vi "StatisticsOnFITSstacks.vi"() -> ()   [LabVIEW 2011]
panel:
  in  "file (use dialog)":path=path "C:/Users/christian/Desktop/tango-signaleSIM.txt"
  out "concatenated string":string="E:\\Auswertung_ISS\\data\\002_2018-06-21_16-44-14\\raw_I000_X0_C0.fits.SIM.fits, 1.293519E+0, 2.813395E+0, 3.203675E-2, 0.000000E+0, 5.713888E+2\r\nE:\\Auswertung_ISS\\data\\002_2018-06-21_16-44-14\\raw_I000_X0_C1.fits.SIM.fits, 5.156106E+0, 1.029898E+1, 3.548476E-1, 0.000000E+0, 1.040870E+3\r\nE:\\Auswertung_ISS\\data\\002_2018-06-21_16-44-14\\raw_I000_X0_C3.fits.SIM.fits, 4.121879E+0, 7.055258E+0, 2.127021E-1, 0.000000E+0, 5.426572E+2\r\nE:\\Auswertung_ISS\\data\\002_2018-06-21_16-44-14\\raw_I000_X1_C0.fits.SIM.fits, 1.210145E+0, 2.047290E+0, -9.516930E-3, 0.000000E+0, 2.892630E+2\r\nE:\\Auswertung_ISS\\data\\002_2018-06-21_16-44-14\\raw_I000_X1_C3.fits.SIM.fits, 1.346602E+0, 2.369957E+0, -2.971059E-2, 0.000000E+0, 2.189330E+2\r\nE:\\Auswertung_ISS\\data\\003_2018-07-03_15-08-29\\raw_I000_X0_C0.fits.SIM.fits, 1.338123E+0, 2.747078E+0, -2.947819E-2, 0.000000E+0, 9.794098E+2\r\nE:\\Auswertung_ISS\\data\\003_2018-07-03_15-08-29\\raw_I000_X0_C1.fits.SIM.fits, 3.859661E+0, 8.027792E+0, -2.797096E-1, 0.000000E+0, 7.325175E+2\r\nE:\\Auswertung_ISS\\data\\003_2018-07-03_15-08-29\\raw_I000_X0_C3.fits.SIM.fits, 2.238438E+0, 3.776091E+0, -1.215679E-1, 0.000000E+0, 6.079381E+2\r\nE:\\Auswertung_ISS\\data\\003_2018-07-03_15-08-29\\raw_I000_X1_C0.fits.SIM.fits, 1.522831E+0, 2.640957E+0, -6.579430E-3, 0.000000E+0, 7.584379E+2\r\nE:\\Auswertung_ISS\\data\\003_2018-07-03_15-08-29\\raw_I000_X1_C3.fits.SIM.fits, 1.066429E+0, 2.187258E+0, 8.379865E-3, 0.000000E+0, 5.129649E+2\r\nE:\\Auswertung_ISS\\data\\003_2018-07-03_15-08-29\\raw_I001_X1_C0.fits.SIM.fits, 1.376409E+0, 2.223739E+0, -6.037710E-3, 0.000000E+0, 5.685716E+2\r\nE:\\Auswertung_ISS\\data\\003_2018-07-03_15-08-29\\raw_I001_X1_C3.fits.SIM.fits, 9.524613E-1, 1.817422E+0, 4.163195E-3, 0.000000E+0, 6.636672E+2\r\nE:\\Auswertung_ISS\\data\\003_2018-07-03_15-08-29\\raw_I002_X1_C0.fits.SIM.fits, 1.321902E+0, 2.089704E+0, -8.378804E-3, 0.000000E+0, 7.800291E+2\r\nE:\\Auswertung_ISS\\data\\003_2018-07-03_15-08-29\\raw_I002_X1_C3.fits.SIM.fits, 9.022409E-1, 1.645853E+0, -5.385981E-3, 0.000000E+0, 8.949173E+2\r\nE:\\Auswertung_ISS\\data\\003_2018-07-03_15-08-29\\raw_I003_X1_C0.fits.SIM.fits, 1.288627E+0, 1.993243E+0, -1.267377E-2, 0.000000E+0, 5.885883E+2\r\nE:\\Auswertung_ISS\\data\\003_2018-07-03_15-08-29\\raw_I003_X1_C3.fits.SIM.fits, 8.580835E-1, 1.470445E+0, -1.397096E-2, 0.000000E+0, 1.369498E+3\r\nE:\\Auswertung_ISS\\data\\003_2018-07-03_15-08-29\\raw_I004_X1_C0.fits.SIM.fits, 1.244456E+0, 1.891138E+0, -1.474137E-2, 0.000000E+0, 8.155282E+2\r\nE:\\Auswertung_ISS\\data\\003_2018-07-03_15-08-29\\raw_I004_X1_C3.fits.SIM.fits, 7.920791E-1, 1.279965E+0, -1.287860E-2, 0.000000E+0, 9.381859E+2\r\nE:\\Auswertung_ISS\\data\\003_2018-07-03_15-08-29\\raw_I005_X1_C0.fits.SIM.fits, 1.217874E+0, 1.802349E+0, -1.420018E-2, 0.000000E+0, 7.741145E+2\r\nE:\\Auswertung_ISS\\data\\003_2018-07-03_15-08-29\\raw_I005_X1_C3.fits.SIM.fits, 7.460330E-1, 1.147673E+0, -9.173622E-3, 0.000000E+0, 6.827392E+2\r\nE:\\Auswertung_ISS\\data\\003_2018-07-03_15-08-29\\raw_I006_X1_C0.fits.SIM.fits, 1.196925E+0, 1.725176E+0, -1.303407E-2, 0.000000E+0, 3.640719E+2\r\nE:\\Auswertung_ISS\\data\\003_2018-07-03_15-08-29\\raw_I006_X1_C3.fits.SIM.fits, 7.214212E-1, 1.099456E+0, -7.464411E-3, 0.000000E+0, 2.052355E+3\r\nE:\\Auswertung_ISS\\data\\003_2018-07-03_15-08-29\\raw_I007_X1_C0.fits.SIM.fits, 1.184295E+0, 1.684428E+0, -1.213101E-2, 0.000000E+0, 3.740072E+2\r\nE:\\Auswertung_ISS\\data\\003_2018-07-03_15-08-29\\raw_I007_X1_C3.fits.SIM.fits, 7.082895E-1, 1.060245E+0, -6.374558E-3, 0.000000E+0, 1.029119E+3\r\nE:\\Auswertung_ISS\\data\\003_2018-07-03_15-08-29\\raw_I008_X1_C0.fits.SIM.fits, 1.178256E+0, 1.672969E+0, -1.182940E-2, 0.000000E+0, 7.563615E+2\r\nE:\\Auswertung_ISS\\data\\003_2018-07-03_15-08-29\\raw_I008_X1_C3.fits.SIM.fits, 7.006131E-1, 1.045075E+0, -5.954691E-3, 0.000000E+0, 1.337770E+3\r\nE:\\Auswertung_ISS\\data\\003_2018-07-03_15-08-29\\raw_I009_X0_C0.fits.SIM.fits, 1.216490E+0, 2.542340E+0, -2.450155E-2, 0.000000E+0, 7.565395E+2\r\nE:\\Auswertung_ISS\\data\\003_2018-07-03_15-08-29\\raw_I009_X0_C1.fits.SIM.fits, 3.969645E+0, 8.299880E+0, -3.314994E-1, 0.000000E+0, 9.914262E+2\r\nE:\\Auswertung_ISS\\data\\003_2018-07-03_15-08-29\\raw_I009_X0_C3.fits.SIM.fits, 1.936800E+0, 3.176954E+0, -1.136370E-1, 0.000000E+0, 6.554843E+2\r\nE:\\Auswertung_ISS\\data\\003_2018-07-03_15-08-29\\raw_I009_X1_C0.fits.SIM.fits, 1.151698E+2, 2.053238E+3, 6.473798E+1, 0.000000E+0, 4.964122E+6\r\nE:\\Auswertung_ISS\\data\\003_2018-07-03_15-08-29\\raw_I009_X1_C3.fits.SIM.fits, 1.220527E+3, 1.606567E+4, 6.178774E+2, 0.000000E+0, 2.381387E+7\r\nE:\\Auswertung_ISS\\data\\004_2018-07-03_17-33-15\\raw_I000_X0_C0.fits.SIM.fits, 1.178057E+0, 2.387788E+0, -2.293336E-2, 0.000000E+0, 3.530892E+2\r\nE:\\Auswertung_ISS\\data\\004_2018-07-03_17-33-15\\raw_I000_X0_C1.fits.SIM.fits, 3.207769E+0, 6.773418E+0, -1.955297E-1, 0.000000E+0, 1.686196E+3\r\nE:\\Auswertung_ISS\\data\\004_2018-07-03_17-33-15\\raw_I000_X0_C3.fits.SIM.fits, 1.521199E+0, 2.480720E+0, -5.475838E-2, 0.000000E+0, 3.812462E+2\r\nE:\\Auswertung_ISS\\data\\004_2018-07-03_17-33-15\\raw_I000_X1_C0.fits.SIM.fits, 1.207292E+0, 1.949696E+0, -5.863263E-3, 0.000000E+0, 8.527518E+2\r\nE:\\Auswertung_ISS\\data\\004_2018-07-03_17-33-15\\raw_I000_X1_C3.fits.SIM.fits, 7.241709E-1, 1.295861E+0, 8.837919E-4, 0.000000E+0, 1.748222E+3\r\nE:\\Auswertung_ISS\\data\\004_2018-07-03_17-33-15\\raw_I001_X1_C0.fits.SIM.fits, 1.169572E+0, 1.829014E+0, -5.958593E-3, 0.000000E+0, 5.068069E+2\r\nE:\\Auswertung_ISS\\data\\004_2018-07-03_17-33-15\\raw_I001_X1_C3.fits.SIM.fits, 7.097706E-1, 1.163805E+0, -2.180760E-4, 0.000000E+0, 1.272369E+3\r\nE:\\Auswertung_ISS\\data\\004_2018-07-03_17-33-15\\raw_I002_X1_C0.fits.SIM.fits, 1.153690E+0, 1.775655E+0, -6.165336E-3, 0.000000E+0, 8.572842E+2\r\nE:\\Auswertung_ISS\\data\\004_2018-07-03_17-33-15\\raw_I002_X1_C3.fits.SIM.fits, 6.968903E-1, 1.093959E+0, -9.725231E-4, 0.000000E+0, 5.995302E+2\r\nE:\\Auswertung_ISS\\data\\004_2018-07-03_17-33-15\\raw_I003_X1_C0.fits.SIM.fits, 1.143082E+0, 1.745283E+0, -6.109823E-3, 0.000000E+0, 8.502672E+2\r\nE:\\Auswertung_ISS\\data\\004_2018-07-03_17-33-15\\raw_I003_X1_C3.fits.SIM.fits, 6.854192E-1, 1.067064E+0, -1.198857E-3, 0.000000E+0, 6.685107E+2\r\nE:\\Auswertung_ISS\\data\\004_2018-07-03_17-33-15\\raw_I004_X1_C0.fits.SIM.fits, 1.133617E+0, 1.709983E+0, -6.070233E-3, 0.000000E+0, 5.567000E+2\r\nE:\\Auswertung_ISS\\data\\004_2018-07-03_17-33-15\\raw_I004_X1_C3.fits.SIM.fits, 6.757222E-1, 1.036550E+0, -1.148639E-3, 0.000000E+0, 8.245127E+2\r\nE:\\Auswertung_ISS\\data\\004_2018-07-03_17-33-15\\raw_I005_X1_C0.fits.SIM.fits, 1.124385E+0, 1.650913E+0, -6.445620E-3, 0.000000E+0, 1.047790E+3\r\nE:\\Auswertung_ISS\\data\\004_2018-07-03_17-33-15\\raw_I005_X1_C3.fits.SIM.fits, 6.672083E-1, 1.008144E+0, -1.706395E-3, 0.000000E+0, 1.310684E+3\r\nE:\\Auswertung_ISS\\data\\004_2018-07-03_17-33-15\\raw_I006_X1_C0.fits.SIM.fits, 1.118813E+0, 1.641358E+0, -6.489867E-3, 0.000000E+0, 5.621022E+2\r\nE:\\Auswertung_ISS\\data\\004_2018-07-03_17-33-15\\raw_I006_X1_C3.fits.SIM.fits, 6.614291E-1, 9.921280E-1, -1.909784E-3, 0.000000E+0, 1.047368E+3\r\nE:\\Auswertung_ISS\\data\\004_2018-07-03_17-33-15\\raw_I007_X1_C0.fits.SIM.fits, 1.113078E+0, 1.626524E+0, -6.676457E-3, 0.000000E+0, 6.429068E+2\r\nE:\\Auswertung_ISS\\data\\004_2018-07-03_17-33-15\\raw_I007_X1_C3.fits.SIM.fits, 6.557754E-1, 9.745117E-1, -2.120740E-3, 0.000000E+0, 7.079556E+2\r\nE:\\Auswertung_ISS\\data\\004_2018-07-03_17-33-15\\raw_I008_X1_C0.fits.SIM.fits, 1.106670E+0, 1.609972E+0, -6.478068E-3, 0.000000E+0, 5.270333E+2\r\nE:\\Auswertung_ISS\\data\\004_2018-07-03_17-33-15\\raw_I008_X1_C3.fits.SIM.fits, 6.534819E-1, 9.693815E-1, -1.453581E-3, 0.000000E+0, 6.050910E+2\r\nE:\\Auswertung_ISS\\data\\004_2018-07-03_17-33-15\\raw_I009_X1_C0.fits.SIM.fits, 1.103888E+0, 1.608102E+0, -6.673347E-3, 0.000000E+0, 7.272290E+2\r\nE:\\Auswertung_ISS\\data\\004_2018-07-03_17-33-15\\raw_I009_X1_C3.fits.SIM.fits, 6.520411E-1, 9.801836E-1, -1.973502E-3, 0.000000E+0, 7.507390E+2\r\nE:\\Auswertung_ISS\\data\\004_2018-07-03_17-33-15\\raw_I010_X1_C0.fits.SIM.fits, 1.099766E+0, 1.593314E+0, -6.739226E-3, 0.000000E+0, 6.720167E+2\r\nE:\\Auswertung_ISS\\data\\004_2018-07-03_17-33-15\\raw_I010_X1_C3.fits.SIM.fits, 6.444918E-1, 9.767788E-1, -1.939564E-3, 0.000000E+0, 6.929294E+2\r\nE:\\Auswertung_ISS\\data\\004_2018-07-03_17-33-15\\raw_I011_X1_C0.fits.SIM.fits, 1.098232E+0, 1.590663E+0, -6.803889E-3, 0.000000E+0, 6.297327E+2\r\nE:\\Auswertung_ISS\\data\\004_2018-07-03_17-33-15\\raw_I011_X1_C3.fits.SIM.fits, 6.416938E-1, 9.659073E-1, -2.201290E-3, 0.000000E+0, 1.132601E+3\r\nE:\\Auswertung_ISS\\data\\004_2018-07-03_17-33-15\\raw_I012_X1_C0.fits.SIM.fits, 1.094868E+0, 1.581222E+0, -6.771624E-3, 0.000000E+0, 6.924265E+2\r\nE:\\Auswertung_ISS\\data\\004_2018-07-03_17-33-15\\raw_I012_X1_C3.fits.SIM.fits, 6.348257E-1, 9.330733E-1, -2.023490E-3, 0.000000E+0, 1.007330E+3\r\nE:\\Auswertung_ISS\\data\\004_2018-07-03_17-33-15\\raw_I013_X1_C0.fits.SIM.fits, 1.091418E+0, 1.572815E+0, -6.660544E-3, 0.000000E+0, 8.789351E+2\r\nE:\\Auswertung_ISS\\data\\004_2018-07-03_17-33-15\\raw_I013_X1_C3.fits.SIM.fits, 6.288961E-1, 9.195451E-1, -1.885985E-3, 0.000000E+0, 1.165087E+3\r\nE:\\Auswertung_ISS\\data\\004_2018-07-03_17-33-15\\raw_I014_X1_C0.fits.SIM.fits, 1.088608E+0, 1.572637E+0, -6.572176E-3, 0.000000E+0, 7.930138E+2\r\nE:\\Auswertung_ISS\\data\\004_2018-07-03_17-33-15\\raw_I014_X1_C3.fits.SIM.fits, 6.240145E-1, 9.116531E-1, -1.725730E-3, 0.000000E+0, 9.153251E+2\r\nE:\\Auswertung_ISS\\data\\004_2018-07-03_17-33-15\\raw_I015_X1_C0.fits.SIM.fits, 1.084505E+0, 1.558305E+0, -6.505683E-3, 0.000000E+0, 4.014997E+2\r\nE:\\Auswertung_ISS\\data\\004_2018-07-03_17-33-15\\raw_I015_X1_C3.fits.SIM.fits, 6.178792E-1, 9.008335E-1, -1.617021E-3, 0.000000E+0, 1.074420E+3\r\nE:\\Auswertung_ISS\\data\\004_2018-07-03_17-33-15\\raw_I016_X1_C0.fits.SIM.fits, 1.083422E+0, 1.556624E+0, -6.624974E-3, 0.000000E+0, 3.853266E+2\r\nE:\\Auswertung_ISS\\data\\004_2018-07-03_17-33-15\\raw_I016_X1_C3.fits.SIM.fits, 6.142787E-1, 9.021998E-1, -1.622850E-3, 0.000000E+0, 8.832935E+2\r\nE:\\Auswertung_ISS\\data\\004_2018-07-03_17-33-15\\raw_I017_X1_C0.fits.SIM.fits, 1.241818E+0, 1.898849E+0, -1.011896E-2, 0.000000E+0, 6.071580E+2\r\nE:\\Auswertung_ISS\\data\\004_2018-07-03_17-33-15\\raw_I017_X1_C3.fits.SIM.fits, 6.135428E-1, 9.080176E-1, -2.219069E-3, 0.000000E+0, 1.471575E+3\r\nE:\\Auswertung_ISS\\data\\005_2018-07-04_08-02-54\\raw_I000_X0_C0.fits.SIM.fits, 1.168267E+0, 2.392403E+0, -2.321325E-2, 0.000000E+0, 5.743918E+2\r\nE:\\Auswertung_ISS\\data\\005_2018-07-04_08-02-54\\raw_I000_X0_C1.fits.SIM.fits, 3.042382E+0, 6.318101E+0, -1.780247E-1, 0.000000E+0, 1.179049E+3\r\nE:\\Auswertung_ISS\\data\\005_2018-07-04_08-02-54\\raw_I000_X0_C3.fits.SIM.fits, 1.098923E+0, 1.709743E+0, -2.960586E-2, 0.000000E+0, 3.829828E+2\r\nE:\\Auswertung_ISS\\data\\005_2018-07-04_08-02-54\\raw_I000_X1_C0.fits.SIM.fits, 1.228053E+0, 1.853084E+0, -9.042175E-3, 0.000000E+0, 4.665842E+2\r\nE:\\Auswertung_ISS\\data\\005_2018-07-04_08-02-54\\raw_I000_X1_C3.fits.SIM.fits, 5.740621E-1, 8.157131E-1, -1.532513E-3, 0.000000E+0, 9.479493E+2\r\nE:\\Auswertung_ISS\\data\\005_2018-07-04_08-02-54\\raw_I001_X1_C0.fits.SIM.fits, 1.166965E+0, 1.716451E+0, -7.717278E-3, 0.000000E+0, 1.209727E+3\r\nE:\\Auswertung_ISS\\data\\005_2018-07-04_08-02-54\\raw_I001_X1_C3.fits.SIM.fits, 5.649782E-1, 8.012455E-1, -1.272490E-3, 0.000000E+0, 1.392420E+3\r\nE:\\Auswertung_ISS\\data\\005_2018-07-04_08-02-54\\raw_I002_X1_C0.fits.SIM.fits, 1.147424E+0, 1.703185E+0, -7.049788E-3, 0.000000E+0, 4.221453E+2\r\nE:\\Auswertung_ISS\\data\\005_2018-07-04_08-02-54\\raw_I002_X1_C3.fits.SIM.fits, 5.609546E-1, 7.931188E-1, -1.130987E-3, 0.000000E+0, 9.405351E+2\r\nE:\\Auswertung_ISS\\data\\005_2018-07-04_08-02-54\\raw_I003_X1_C0.fits.SIM.fits, 1.126167E+0, 1.636829E+0, -7.009850E-3, 0.000000E+0, 7.209102E+2\r\nE:\\Auswertung_ISS\\data\\005_2018-07-04_08-02-54\\raw_I003_X1_C3.fits.SIM.fits, 5.537584E-1, 7.808799E-1, -7.431867E-4, 0.000000E+0, 1.088224E+3\r\nE:\\Auswertung_ISS\\data\\005_2018-07-04_08-02-54\\raw_I004_X1_C0.fits.SIM.fits, 1.113321E+0, 1.610422E+0, -6.982198E-3, 0.000000E+0, 3.967598E+2\r\nE:\\Auswertung_ISS\\data\\005_2018-07-04_08-02-54\\raw_I004_X1_C3.fits.SIM.fits, 5.514046E-1, 7.721213E-1, -7.544226E-4, 0.000000E+0, 8.216857E+2\r\nE:\\Auswertung_ISS\\data\\005_2018-07-04_08-02-54\\raw_I005_X1_C0.fits.SIM.fits, 1.103067E+0, 1.593565E+0, -6.857917E-3, 0.000000E+0, 4.775246E+2\r\nE:\\Auswertung_ISS\\data\\005_2018-07-04_08-02-54\\raw_I005_X1_C3.fits.SIM.fits, 5.486360E-1, 7.665561E-1, -6.179845E-4, 0.000000E+0, 5.884370E+2\r\nE:\\Auswertung_ISS\\data\\005_2018-07-04_08-02-54\\raw_I006_X1_C0.fits.SIM.fits, 1.093904E+0, 1.570558E+0, -6.920714E-3, 0.000000E+0, 6.544910E+2\r\nE:\\Auswertung_ISS\\data\\005_2018-07-04_08-02-54\\raw_I006_X1_C3.fits.SIM.fits, 5.464946E-1, 7.668871E-1, -6.099782E-4, 0.000000E+0, 1.330119E+3\r\nE:\\Auswertung_ISS\\data\\005_2018-07-04_08-02-54\\raw_I007_X1_C0.fits.SIM.fits, 1.087188E+0, 1.564195E+0, -6.751027E-3, 0.000000E+0, 5.254551E+2\r\nE:\\Auswertung_ISS\\data\\005_2018-07-04_08-02-54\\raw_I007_X1_C3.fits.SIM.fits, 5.451777E-1, 7.614440E-1, -5.663460E-4, 0.000000E+0, 9.518828E+2\r\nE:\\Auswertung_ISS\\data\\005_2018-07-04_08-02-54\\raw_I008_X1_C0.fits.SIM.fits, 1.079745E+0, 1.542835E+0, -6.759820E-3, 0.000000E+0, 4.754071E+2\r\nE:\\Auswertung_ISS\\data\\005_2018-07-04_08-02-54\\raw_I008_X1_C3.fits.SIM.fits, 5.436806E-1, 7.669905E-1, -6.040051E-4, 0.000000E+0, 1.077933E+3\r\nE:\\Auswertung_ISS\\data\\005_2018-07-04_08-02-54\\raw_I009_X1_C0.fits.SIM.fits, 1.075054E+0, 1.537219E+0, -6.715304E-3, 0.000000E+0, 1.070141E+3\r\nE:\\Auswertung_ISS\\data\\005_2018-07-04_08-02-54\\raw_I009_X1_C3.fits.SIM.fits, 5.419445E-1, 7.547276E-1, -6.042233E-4, 0.000000E+0, 1.172648E+3\r\nE:\\Auswertung_ISS\\data\\005_2018-07-04_08-02-54\\raw_I010_X1_C0.fits.SIM.fits, 1.071120E+0, 1.528894E+0, -6.637398E-3, 0.000000E+0, 6.953884E+2\r\nE:\\Auswertung_ISS\\data\\005_2018-07-04_08-02-54\\raw_I010_X1_C3.fits.SIM.fits, 5.398463E-1, 7.559122E-1, -5.406494E-4, 0.000000E+0, 1.200631E+3\r\nE:\\Auswertung_ISS\\data\\005_2018-07-04_08-02-54\\raw_I011_X1_C0.fits.SIM.fits, 1.066154E+0, 1.515149E+0, -6.609291E-3, 0.000000E+0, 4.025648E+2\r\nE:\\Auswertung_ISS\\data\\005_2018-07-04_08-02-54\\raw_I011_X1_C3.fits.SIM.fits, 5.381187E-1, 7.581280E-1, -4.396083E-4, 0.000000E+0, 1.214015E+3\r\nE:\\Auswertung_ISS\\data\\005_2018-07-04_08-02-54\\raw_I012_X1_C0.fits.SIM.fits, 1.062224E+0, 1.514587E+0, -6.448907E-3, 0.000000E+0, 6.856676E+2\r\nE:\\Auswertung_ISS\\data\\005_2018-07-04_08-02-54\\raw_I012_X1_C3.fits.SIM.fits, 5.366250E-1, 7.576223E-1, -3.866185E-4, 0.000000E+0, 1.015641E+3\r\nE:\\Auswertung_ISS\\data\\005_2018-07-04_08-02-54\\raw_I013_X1_C0.fits.SIM.fits, 1.057811E+0, 1.501086E+0, -6.549502E-3, 0.000000E+0, 8.431631E+2\r\nE:\\Auswertung_ISS\\data\\005_2018-07-04_08-02-54\\raw_I013_X1_C3.fits.SIM.fits, 5.350741E-1, 7.434772E-1, -3.976152E-4, 0.000000E+0, 1.028520E+3\r\nE:\\Auswertung_ISS\\data\\005_2018-07-04_08-02-54\\raw_I014_X1_C0.fits.SIM.fits, 1.055553E+0, 1.498822E+0, -6.397800E-3, 0.000000E+0, 5.896923E+2\r\nE:\\Auswertung_ISS\\data\\005_2018-07-04_08-02-54\\raw_I014_X1_C3.fits.SIM.fits, 5.333580E-1, 7.450038E-1, -3.825911E-4, 0.000000E+0, 9.034543E+2\r\nE:\\Auswertung_ISS\\data\\005_2018-07-04_08-02-54\\raw_I015_X1_C0.fits.SIM.fits, 1.051548E+0, 1.486582E+0, -6.435934E-3, 0.000000E+0, 2.464364E+2\r\nE:\\Auswertung_ISS\\data\\005_2018-07-04_08-02-54\\raw_I015_X1_C3.fits.SIM.fits, 5.313362E-1, 7.351835E-1, -3.081133E-4, 0.000000E+0, 8.765760E+2\r\nE:\\Auswertung_ISS\\data\\005_2018-07-04_08-02-54\\raw_I016_X1_C0.fits.SIM.fits, 1.047979E+0, 1.483462E+0, -6.301912E-3, 0.000000E+0, 4.212937E+2\r\nE:\\Auswertung_ISS\\data\\005_2018-07-04_08-02-54\\raw_I016_X1_C3.fits.SIM.fits, 5.303586E-1, 7.424460E-1, -3.963325E-4, 0.000000E+0, 1.428170E+3\r\nE:\\Auswertung_ISS\\data\\006_2018-07-04_15-43-18\\raw_I000_X0_C0.fits.SIM.fits, 1.173188E+0, 2.418540E+0, -2.354629E-2, 0.000000E+0, 4.402941E+2\r\nE:\\Auswertung_ISS\\data\\006_2018-07-04_15-43-18\\raw_I000_X0_C1.fits.SIM.fits, 2.924494E+0, 6.028345E+0, -1.636071E-1, 0.000000E+0, 9.315766E+2\r\nE:\\Auswertung_ISS\\data\\006_2018-07-04_15-43-18\\raw_I000_X0_C3.fits.SIM.fits, 9.369917E-1, 1.419599E+0, -1.991960E-2, 0.000000E+0, 6.888892E+2\r\nE:\\Auswertung_ISS\\data\\006_2018-07-04_15-43-18\\raw_I000_X1_C0.fits.SIM.fits, 1.167226E+0, 1.601891E+0, -1.181800E-2, 0.000000E+0, 5.933480E+2\r\nE:\\Auswertung_ISS\\data\\006_2018-07-04_15-43-18\\raw_I000_X1_C3.fits.SIM.fits, 5.161158E-1, 7.151016E-1, -4.825938E-4, 0.000000E+0, 1.697749E+3\r\nE:\\Auswertung_ISS\\data\\006_2018-07-04_15-43-18\\raw_I001_X1_C0.fits.SIM.fits, 1.116488E+0, 1.530844E+0, -9.946897E-3, 0.000000E+0, 6.367750E+2\r\nE:\\Auswertung_ISS\\data\\006_2018-07-04_15-43-18\\raw_I001_X1_C3.fits.SIM.fits, 5.154800E-1, 7.122431E-1, -6.673413E-4, 0.000000E+0, 1.607819E+3\r\nE:\\Auswertung_ISS\\data\\006_2018-07-04_15-43-18\\raw_I002_X1_C0.fits.SIM.fits, 1.098814E+0, 1.505064E+0, -9.540462E-3, 0.000000E+0, 2.874549E+2\r\nE:\\Auswertung_ISS\\data\\006_2018-07-04_15-43-18\\raw_I002_X1_C3.fits.SIM.fits, 5.132112E-1, 7.099640E-1, -5.868003E-4, 0.000000E+0, 1.146126E+3\r\nE:\\Auswertung_ISS\\data\\006_2018-07-04_15-43-18\\raw_I003_X1_C0.fits.SIM.fits, 1.087255E+0, 1.488291E+0, -9.129129E-3, 0.000000E+0, 3.591404E+2\r\nE:\\Auswertung_ISS\\data\\006_2018-07-04_15-43-18\\raw_I003_X1_C3.fits.SIM.fits, 5.118757E-1, 7.201306E-1, -5.091988E-4, 0.000000E+0, 1.603813E+3\r\nE:\\Auswertung_ISS\\data\\007_2018-07-04_16-44-22\\raw_I000_X0_C0.fits.SIM.fits, 1.153519E+0, 2.645130E+0, 2.393591E-2, 0.000000E+0, 3.971248E+2\r\nE:\\Auswertung_ISS\\data\\007_2018-07-04_16-44-22\\raw_I000_X0_C1.fits.SIM.fits, 3.857970E+0, 7.510054E+0, 6.305399E-2, 0.000000E+0, 9.667203E+2\r\nE:\\Auswertung_ISS\\data\\007_2018-07-04_16-44-22\\raw_I000_X0_C3.fits.SIM.fits, 1.023600E+0, 1.481754E+0, 4.806154E-3, 0.000000E+0, 2.218139E+2\r\nE:\\Auswertung_ISS\\data\\007_2018-07-04_16-44-22\\raw_I000_X1_C0.fits.SIM.fits, 1.196240E+0, 1.789233E+0, -7.721109E-3, 0.000000E+0, 2.244067E+2\r\nE:\\Auswertung_ISS\\data\\007_2018-07-04_16-44-22\\raw_I000_X1_C3.fits.SIM.fits, 5.829489E-1, 8.366924E-1, -8.507837E-4, 0.000000E+0, 9.379310E+2\r\nE:\\Auswertung_ISS\\data\\007_2018-07-04_16-44-22\\raw_I001_X1_C0.fits.SIM.fits, 1.138294E+0, 1.672213E+0, -6.483374E-3, 0.000000E+0, 5.219246E+2\r\nE:\\Auswertung_ISS\\data\\007_2018-07-04_16-44-22\\raw_I001_X1_C3.fits.SIM.fits, 5.742043E-1, 8.091986E-1, -7.224752E-4, 0.000000E+0, 6.994556E+2\r\nE:\\Auswertung_ISS\\data\\007_2018-07-04_16-44-22\\raw_I002_X1_C0.fits.SIM.fits, 1.117667E+0, 1.610874E+0, -5.967891E-3, 0.000000E+0, 6.300037E+2\r\nE:\\Auswertung_ISS\\data\\007_2018-07-04_16-44-22\\raw_I002_X1_C3.fits.SIM.fits, 5.677322E-1, 7.945078E-1, -4.561589E-4, 0.000000E+0, 6.261265E+2\r\nE:\\Auswertung_ISS\\data\\007_2018-07-04_16-44-22\\raw_I003_X1_C0.fits.SIM.fits, 1.104924E+0, 1.613847E+0, -5.905481E-3, 0.000000E+0, 6.381712E+2\r\nE:\\Auswertung_ISS\\data\\007_2018-07-04_16-44-22\\raw_I003_X1_C3.fits.SIM.fits, 5.665135E-1, 8.095917E-1, -4.370291E-4, 0.000000E+0, 9.460343E+2\r\nE:\\Auswertung_ISS\\data\\007_2018-07-04_16-44-22\\raw_I004_X1_C0.fits.SIM.fits, 1.094761E+0, 1.586387E+0, -5.725719E-3, 0.000000E+0, 4.823523E+2\r\nE:\\Auswertung_ISS\\data\\007_2018-07-04_16-44-22\\raw_I004_X1_C3.fits.SIM.fits, 5.646007E-1, 8.049347E-1, -3.713122E-4, 0.000000E+0, 9.834833E+2\r\nE:\\Auswertung_ISS\\data\\007_2018-07-04_16-44-22\\raw_I005_X1_C0.fits.SIM.fits, 1.086430E+0, 1.550623E+0, -5.757585E-3, 0.000000E+0, 7.921680E+2\r\nE:\\Auswertung_ISS\\data\\007_2018-07-04_16-44-22\\raw_I005_X1_C3.fits.SIM.fits, 5.622428E-1, 7.931760E-1, -1.688326E-4, 0.000000E+0, 1.029930E+3\r\nE:\\Auswertung_ISS\\data\\007_2018-07-04_16-44-22\\raw_I006_X1_C0.fits.SIM.fits, 1.080670E+0, 1.556944E+0, -5.527289E-3, 0.000000E+0, 4.178517E+2\r\nE:\\Auswertung_ISS\\data\\007_2018-07-04_16-44-22\\raw_I006_X1_C3.fits.SIM.fits, 5.617751E-1, 7.960590E-1, -7.710413E-5, 0.000000E+0, 9.626111E+2\r\nE:\\Auswertung_ISS\\data\\007_2018-07-04_16-44-22\\raw_I007_X1_C0.fits.SIM.fits, 1.073678E+0, 1.525147E+0, -5.556067E-3, 0.000000E+0, 5.914534E+2\r\nE:\\Auswertung_ISS\\data\\007_2018-07-04_16-44-22\\raw_I007_X1_C3.fits.SIM.fits, 5.592173E-1, 7.789348E-1, -4.470449E-6, 0.000000E+0, 5.747207E+2\r\nE:\\Auswertung_ISS\\data\\007_2018-07-04_16-44-22\\raw_I008_X1_C0.fits.SIM.fits, 1.070393E+0, 1.532612E+0, -5.517926E-3, 0.000000E+0, 6.460666E+2\r\nE:\\Auswertung_ISS\\data\\007_2018-07-04_16-44-22\\raw_I008_X1_C3.fits.SIM.fits, 5.584064E-1, 7.797402E-1, -1.403181E-5, 0.000000E+0, 4.066313E+2\r\nE:\\Auswertung_ISS\\data\\007_2018-07-04_16-44-22\\raw_I008_X1_C3.fits.simpleSIM.fits, 9.756062E-1, 5.934669E-1, -1.062698E-3, 3.518001E-2, 4.811809E+2\r\nE:\\Auswertung_ISS\\data\\007_2018-07-04_16-44-22\\raw_I009_X1_C0.fits.SIM.fits, 1.064844E+0, 1.507894E+0, -5.596534E-3, 0.000000E+0, 4.210096E+2\r\nE:\\Auswertung_ISS\\data\\007_2018-07-04_16-44-22\\raw_I009_X1_C3.fits.SIM.fits, 5.560395E-1, 7.785271E-1, -1.746596E-5, 0.000000E+0, 1.219767E+3\r\nE:\\Auswertung_ISS\\data\\007_2018-07-04_16-44-22\\raw_I010_X1_C0.fits.SIM.fits, 1.062220E+0, 1.504640E+0, -5.459205E-3, 0.000000E+0, 6.228591E+2\r\nE:\\Auswertung_ISS\\data\\007_2018-07-04_16-44-22\\raw_I010_X1_C3.fits.SIM.fits, 5.553953E-1, 7.835472E-1, 5.496466E-5, 0.000000E+0, 1.274058E+3\r\nE:\\Auswertung_ISS\\data\\007_2018-07-04_16-44-22\\raw_I011_X1_C0.fits.SIM.fits, 1.060179E+0, 1.500548E+0, -5.420390E-3, 0.000000E+0, 4.995820E+2\r\nE:\\Auswertung_ISS\\data\\007_2018-07-04_16-44-22\\raw_I011_X1_C3.fits.SIM.fits, 5.544396E-1, 7.838519E-1, 2.043480E-4, 0.000000E+0, 1.140602E+3\r\nE:\\Auswertung_ISS\\data\\007_2018-07-04_16-44-22\\raw_I012_X1_C0.fits.SIM.fits, 1.056946E+0, 1.491268E+0, -5.362876E-3, 0.000000E+0, 3.350965E+2\r\nE:\\Auswertung_ISS\\data\\007_2018-07-04_16-44-22\\raw_I012_X1_C3.fits.SIM.fits, 5.532384E-1, 7.741418E-1, 2.192681E-4, 0.000000E+0, 9.582665E+2\r\nE:\\Auswertung_ISS\\data\\007_2018-07-04_16-44-22\\raw_I013_X1_C0.fits.SIM.fits, 1.054764E+0, 1.495314E+0, -5.343243E-3, 0.000000E+0, 3.678161E+2\r\nE:\\Auswertung_ISS\\data\\007_2018-07-04_16-44-22\\raw_I013_X1_C3.fits.SIM.fits, 5.516079E-1, 7.765394E-1, 1.682077E-4, 0.000000E+0, 1.040956E+3\r\nE:\\Auswertung_ISS\\data\\007_2018-07-04_16-44-22\\raw_I014_X1_C0.fits.SIM.fits, 1.051305E+0, 1.483902E+0, -5.243355E-3, 0.000000E+0, 5.850872E+2\r\nE:\\Auswertung_ISS\\data\\007_2018-07-04_16-44-22\\raw_I014_X1_C3.fits.SIM.fits, 5.500311E-1, 7.715969E-1, 2.253367E-4, 0.000000E+0, 1.121011E+3\r\nE:\\Auswertung_ISS\\data\\007_2018-07-04_16-44-22\\raw_I015_X1_C0.fits.SIM.fits, 1.047873E+0, 1.477831E+0, -5.204884E-3, 0.000000E+0, 4.423718E+2\r\nE:\\Auswertung_ISS\\data\\007_2018-07-04_16-44-22\\raw_I015_X1_C3.fits.SIM.fits, 5.480902E-1, 7.653563E-1, 2.163062E-4, 0.000000E+0, 1.302920E+3\r\nE:\\Auswertung_ISS\\data\\007_2018-07-04_16-44-22\\raw_I016_X1_C0.fits.SIM.fits, 1.047071E+0, 1.487131E+0, -5.224378E-3, 0.000000E+0, 9.012682E+2\r\nE:\\Auswertung_ISS\\data\\007_2018-07-04_16-44-22\\raw_I016_X1_C3.fits.SIM.fits, 5.473597E-1, 7.600744E-1, 1.331081E-4, 0.000000E+0, 5.495349E+2\r\nE:\\Auswertung_ISS\\data\\007_2018-07-04_16-44-22\\raw_I017_X1_C0.fits.SIM.fits, 1.162750E+0, 1.656961E+0, -8.553688E-3, 0.000000E+0, 4.017816E+2\r\nE:\\Auswertung_ISS\\data\\007_2018-07-04_16-44-22\\raw_I017_X1_C3.fits.SIM.fits, 5.456086E-1, 7.595779E-1, -2.192173E-4, 0.000000E+0, 1.091998E+3\r\nE:\\Auswertung_ISS\\data\\008_2018-07-05_08-02-52\\raw_I000_X0_C0.fits.SIM.fits, 1.148379E+0, 2.222971E+0, -1.844273E-2, 0.000000E+0, 3.856597E+2\r\nE:\\Auswertung_ISS\\data\\008_2018-07-05_08-02-52\\raw_I000_X0_C1.fits.SIM.fits, 2.394992E+0, 4.660775E+0, -7.314335E-2, 0.000000E+0, 7.939623E+2\r\nE:\\Auswertung_ISS\\data\\008_2018-07-05_08-02-52\\raw_I000_X0_C3.fits.SIM.fits, 7.212795E-1, 1.039594E+0, -5.723648E-3, 0.000000E+0, 4.026962E+2\r\nE:\\Auswertung_ISS\\data\\008_2018-07-05_08-02-52\\raw_I000_X1_C0.fits.SIM.fits, 1.202009E+0, 1.771153E+0, -8.815809E-3, 0.000000E+0, 4.285009E+2\r\nE:\\Auswertung_ISS\\data\\008_2018-07-05_08-02-52\\raw_I000_X1_C3.fits.SIM.fits, 5.883181E-1, 8.647142E-1, -1.495725E-3, 0.000000E+0, 8.403303E+2\r\nE:\\Auswertung_ISS\\data\\008_2018-07-05_08-02-52\\raw_I001_X1_C0.fits.SIM.fits, 1.141505E+0, 1.658387E+0, -7.034378E-3, 0.000000E+0, 5.092637E+2\r\nE:\\Auswertung_ISS\\data\\008_2018-07-05_08-02-52\\raw_I001_X1_C3.fits.SIM.fits, 5.780757E-1, 8.329380E-1, -1.291502E-3, 0.000000E+0, 7.277889E+2\r\nE:\\Auswertung_ISS\\data\\008_2018-07-05_08-02-52\\raw_I002_X1_C0.fits.SIM.fits, 1.118703E+0, 1.621198E+0, -6.548159E-3, 0.000000E+0, 5.058632E+2\r\nE:\\Auswertung_ISS\\data\\008_2018-07-05_08-02-52\\raw_I002_X1_C3.fits.SIM.fits, 5.729400E-1, 8.195264E-1, -1.049177E-3, 0.000000E+0, 8.910027E+2\r\nE:\\Auswertung_ISS\\data\\008_2018-07-05_08-02-52\\raw_I003_X1_C0.fits.SIM.fits, 1.100937E+0, 1.591233E+0, -6.214834E-3, 0.000000E+0, 5.665538E+2\r\nE:\\Auswertung_ISS\\data\\008_2018-07-05_08-02-52\\raw_I003_X1_C3.fits.SIM.fits, 5.693229E-1, 8.083807E-1, -8.714600E-4, 0.000000E+0, 5.859122E+2\r\nE:\\Auswertung_ISS\\data\\008_2018-07-05_08-02-52\\raw_I004_X1_C0.fits.SIM.fits, 1.088585E+0, 1.569994E+0, -6.116154E-3, 0.000000E+0, 3.472624E+2\r\nE:\\Auswertung_ISS\\data\\008_2018-07-05_08-02-52\\raw_I004_X1_C3.fits.SIM.fits, 5.683783E-1, 8.144570E-1, -8.879215E-4, 0.000000E+0, 9.490573E+2\r\nE:\\Auswertung_ISS\\data\\008_2018-07-05_08-02-52\\raw_I005_X1_C0.fits.SIM.fits, 1.078709E+0, 1.554057E+0, -6.028421E-3, 0.000000E+0, 3.866093E+2\r\nE:\\Auswertung_ISS\\data\\008_2018-07-05_08-02-52\\raw_I005_X1_C3.fits.SIM.fits, 5.661956E-1, 8.063986E-1, -8.135665E-4, 0.000000E+0, 1.206259E+3\r\nE:\\Auswertung_ISS\\data\\008_2018-07-05_08-02-52\\raw_I006_X1_C0.fits.SIM.fits, 1.070579E+0, 1.536859E+0, -5.875261E-3, 0.000000E+0, 3.029638E+2\r\nE:\\Auswertung_ISS\\data\\008_2018-07-05_08-02-52\\raw_I006_X1_C3.fits.SIM.fits, 5.655424E-1, 8.111434E-1, -8.166707E-4, 0.000000E+0, 1.835373E+3\r\nE:\\Auswertung_ISS\\data\\008_2018-07-05_08-02-52\\raw_I007_X1_C0.fits.SIM.fits, 1.064083E+0, 1.528916E+0, -5.805853E-3, 0.000000E+0, 4.198567E+2\r\nE:\\Auswertung_ISS\\data\\008_2018-07-05_08-02-52\\raw_I007_X1_C3.fits.SIM.fits, 5.641893E-1, 8.154879E-1, -7.558414E-4, 0.000000E+0, 1.314626E+3\r\nE:\\Auswertung_ISS\\data\\008_2018-07-05_08-02-52\\raw_I008_X1_C0.fits.SIM.fits, 1.058198E+0, 1.515109E+0, -5.716312E-3, 0.000000E+0, 3.127709E+2\r\nE:\\Auswertung_ISS\\data\\008_2018-07-05_08-02-52\\raw_I008_X1_C3.fits.SIM.fits, 5.628286E-1, 8.024234E-1, -7.728365E-4, 0.000000E+0, 1.494765E+3\r\nE:\\Auswertung_ISS\\data\\008_2018-07-05_08-02-52\\raw_I009_X1_C0.fits.SIM.fits, 1.053399E+0, 1.508024E+0, -5.628926E-3, 0.000000E+0, 3.604301E+2\r\nE:\\Auswertung_ISS\\data\\008_2018-07-05_08-02-52\\raw_I009_X1_C3.fits.SIM.fits, 5.614796E-1, 8.032793E-1, -7.241538E-4, 0.000000E+0, 1.339423E+3\r\nE:\\Auswertung_ISS\\data\\008_2018-07-05_08-02-52\\raw_I010_X1_C0.fits.SIM.fits, 1.048438E+0, 1.499447E+0, -5.609204E-3, 0.000000E+0, 7.566072E+2\r\nE:\\Auswertung_ISS\\data\\008_2018-07-05_08-02-52\\raw_I010_X1_C3.fits.SIM.fits, 5.598310E-1, 7.975740E-1, -7.201707E-4, 0.000000E+0, 8.480476E+2\r\nE:\\Auswertung_ISS\\data\\008_2018-07-05_08-02-52\\raw_I011_X1_C0.fits.SIM.fits, 1.044377E+0, 1.490749E+0, -5.590479E-3, 0.000000E+0, 3.436553E+2\r\nE:\\Auswertung_ISS\\data\\008_2018-07-05_08-02-52\\raw_I011_X1_C3.fits.SIM.fits, 5.579582E-1, 7.956876E-1, -7.347059E-4, 0.000000E+0, 1.222693E+3\r\nE:\\Auswertung_ISS\\data\\008_2018-07-05_08-02-52\\raw_I012_X1_C0.fits.SIM.fits, 1.040627E+0, 1.484045E+0, -5.533625E-3, 0.000000E+0, 7.895819E+2\r\nE:\\Auswertung_ISS\\data\\008_2018-07-05_08-02-52\\raw_I012_X1_C3.fits.SIM.fits, 5.563867E-1, 7.798143E-1, -7.386163E-4, 0.000000E+0, 4.880072E+2\r\nE:\\Auswertung_ISS\\data\\008_2018-07-05_08-02-52\\raw_I013_X1_C0.fits.SIM.fits, 1.036955E+0, 1.476465E+0, -5.388023E-3, 0.000000E+0, 6.334623E+2\r\nE:\\Auswertung_ISS\\data\\008_2018-07-05_08-02-52\\raw_I013_X1_C3.fits.SIM.fits, 5.544554E-1, 7.814884E-1, -6.736483E-4, 0.000000E+0, 8.812255E+2\r\nE:\\Auswertung_ISS\\data\\008_2018-07-05_08-02-52\\raw_I014_X1_C0.fits.SIM.fits, 1.035031E+0, 1.476933E+0, -5.406284E-3, 0.000000E+0, 8.390779E+2\r\nE:\\Auswertung_ISS\\data\\008_2018-07-05_08-02-52\\raw_I014_X1_C3.fits.SIM.fits, 5.526023E-1, 7.840290E-1, -6.420569E-4, 0.000000E+0, 1.696114E+3\r\nE:\\Auswertung_ISS\\data\\008_2018-07-05_08-02-52\\raw_I015_X1_C0.fits.SIM.fits, 1.031940E+0, 1.468893E+0, -5.353902E-3, 0.000000E+0, 2.968327E+2\r\nE:\\Auswertung_ISS\\data\\008_2018-07-05_08-02-52\\raw_I015_X1_C3.fits.SIM.fits, 5.507609E-1, 7.733699E-1, -5.823198E-4, 0.000000E+0, 1.089923E+3\r\nE:\\Auswertung_ISS\\data\\008_2018-07-05_08-02-52\\raw_I016_X1_C0.fits.SIM.fits, 1.029475E+0, 1.460240E+0, -5.299052E-3, 0.000000E+0, 5.076005E+2\r\nE:\\Auswertung_ISS\\data\\008_2018-07-05_08-02-52\\raw_I016_X1_C3.fits.SIM.fits, 5.488108E-1, 7.656781E-1, -5.384322E-4, 0.000000E+0, 5.239290E+2\r\nE:\\Auswertung_ISS\\data\\008_2018-07-05_08-02-52\\raw_I017_X1_C0.fits.SIM.fits, 1.143046E+0, 1.650063E+0, -8.704591E-3, 0.000000E+0, 4.047151E+2\r\nE:\\Auswertung_ISS\\data\\008_2018-07-05_08-02-52\\raw_I017_X1_C3.fits.SIM.fits, 5.431783E-1, 7.666736E-1, -8.583751E-4, 0.000000E+0, 1.267076E+3\r\nE:\\Auswertung_ISS\\data\\009_2018-07-05_20-57-36\\raw_I000_X0_C0.fits.SIM.fits, 1.095481E+0, 2.213086E+0, 9.713236E-3, 0.000000E+0, 4.552138E+2\r\nE:\\Auswertung_ISS\\data\\009_2018-07-05_20-57-36\\raw_I000_X0_C1.fits.SIM.fits, 3.820018E+0, 8.163619E+0, 6.830375E-2, 0.000000E+0, 1.048718E+3\r\nE:\\Auswertung_ISS\\data\\009_2018-07-05_20-57-36\\raw_I000_X0_C3.fits.SIM.fits, 2.317444E+0, 4.457747E+0, 1.745774E-2, 0.000000E+0, 6.529139E+2\r\nE:\\Auswertung_ISS\\data\\009_2018-07-05_20-57-36\\raw_I000_X1_C3.fits.SIM.fits, 8.102129E-1, 1.161321E+0, -8.607505E-4, 0.000000E+0, 1.162566E+3\r\nE:\\Auswertung_ISS\\data\\009_2018-07-05_20-57-36\\raw_I001_X1_C3.fits.SIM.fits, 7.880289E-1, 1.109084E+0, -2.994123E-4, 0.000000E+0, 1.143288E+3\r\nE:\\Auswertung_ISS\\data\\009_2018-07-05_20-57-36\\raw_I002_X1_C3.fits.SIM.fits, 7.797577E-1, 1.103446E+0, -1.481503E-4, 0.000000E+0, 1.379730E+3\r\nE:\\Auswertung_ISS\\data\\009_2018-07-05_20-57-36\\raw_I003_X1_C3.fits.SIM.fits, 7.722451E-1, 1.086300E+0, 1.212822E-4, 0.000000E+0, 1.238731E+3\r\nE:\\Auswertung_ISS\\data\\009_2018-07-05_20-57-36\\raw_I004_X1_C3.fits.SIM.fits, 7.669797E-1, 1.076087E+0, 1.388112E-4, 0.000000E+0, 1.660364E+3\r\nE:\\Auswertung_ISS\\data\\009_2018-07-05_20-57-36\\raw_I005_X1_C3.fits.SIM.fits, 7.623354E-1, 1.063843E+0, 2.429270E-4, 0.000000E+0, 1.089695E+3\r\nE:\\Auswertung_ISS\\data\\009_2018-07-05_20-57-36\\raw_I006_X1_C3.fits.SIM.fits, 7.578356E-1, 1.059566E+0, 2.568955E-4, 0.000000E+0, 1.312015E+3\r\nE:\\Auswertung_ISS\\data\\009_2018-07-05_20-57-36\\raw_I007_X1_C3.fits.SIM.fits, 7.537718E-1, 1.054976E+0, 2.752649E-4, 0.000000E+0, 1.390512E+3\r\nE:\\Auswertung_ISS\\data\\009_2018-07-05_20-57-36\\raw_I008_X1_C3.fits.SIM.fits, 7.497759E-1, 1.045071E+0, 2.596070E-4, 0.000000E+0, 1.098528E+3\r\nE:\\Auswertung_ISS\\data\\009_2018-07-05_20-57-36\\raw_I009_X1_C3.fits.SIM.fits, 7.553792E-1, 1.047395E+0, -2.532968E-5, 0.000000E+0, 9.539799E+2\r\nE:\\Auswertung_ISS\\data\\009_2018-07-05_20-57-36\\raw_I010_X1_C3.fits.SIM.fits, 7.448525E-1, 1.035980E+0, -1.396920E-4, 0.000000E+0, 1.466276E+3\r\nE:\\Auswertung_ISS\\data\\009_2018-07-05_20-57-36\\raw_I011_X1_C3.fits.SIM.fits, 7.403386E-1, 1.021841E+0, -3.756509E-5, 0.000000E+0, 1.044579E+3\r\nE:\\Auswertung_ISS\\data\\010_2018-07-06_17-20-26\\raw_I000_X0_C0.fits.SIM.fits, 1.103677E+0, 2.278387E+0, 9.929147E-3, 0.000000E+0, 7.836542E+2\r\nE:\\Auswertung_ISS\\data\\010_2018-07-06_17-20-26\\raw_I000_X0_C1.fits.SIM.fits, 3.551940E+0, 7.390674E+0, 4.617931E-2, 0.000000E+0, 9.348444E+2\r\nE:\\Auswertung_ISS\\data\\010_2018-07-06_17-20-26\\raw_I000_X0_C3.fits.SIM.fits, 1.872104E+0, 3.393058E+0, 7.529059E-3, 0.000000E+0, 6.464011E+2\r\nE:\\Auswertung_ISS\\data\\010_2018-07-06_17-20-26\\raw_I000_X1_C3.fits.SIM.fits, 7.384075E-1, 1.047475E+0, 7.400314E-5, 0.000000E+0, 1.178863E+3\r\nE:\\Auswertung_ISS\\data\\010_2018-07-06_17-20-26\\raw_I001_X0_C0.fits.SIM.fits, 2.097842E+0, 7.191353E+1, NaN, 0.000000E+0, 3.056341E+4\r\nE:\\Auswertung_ISS\\data\\010_2018-07-06_17-20-26\\raw_I001_X0_C1.fits.SIM.fits, 2.207276E-1, 1.665756E+1, NaN, 0.000000E+0, 1.981299E+4\r\nE:\\Auswertung_ISS\\data\\010_2018-07-06_17-20-26\\raw_I001_X0_C3.fits.SIM.fits, 2.093130E+0, 7.869714E+1, NaN, 0.000000E+0, 3.070107E+4\r\nE:\\Auswertung_ISS\\data\\011_2018-07-06_17-40-54\\raw_I000_X0_C0.fits.SIM.fits, 9.329651E-1, 1.827524E+0, 4.917080E-3, 0.000000E+0, 3.218249E+2\r\nE:\\Auswertung_ISS\\data\\011_2018-07-06_17-40-54\\raw_I000_X0_C1.fits.SIM.fits, 3.367464E+0, 7.650311E+0, 2.959199E-2, 0.000000E+0, 9.764470E+2\r\nE:\\Auswertung_ISS\\data\\011_2018-07-06_17-40-54\\raw_I000_X0_C3.fits.SIM.fits, 2.047028E+0, 3.858013E+0, 1.368241E-3, 0.000000E+0, 2.739189E+2\r\nE:\\Auswertung_ISS\\data\\011_2018-07-06_17-40-54\\raw_I000_X1_C3.fits.SIM.fits, 9.367726E-1, 1.327563E+0, 3.956851E-4, 0.000000E+0, 1.508956E+3\r\nE:\\Auswertung_ISS\\data\\011_2018-07-06_17-40-54\\raw_I001_X1_C3.fits.SIM.fits, 9.031187E-1, 1.272661E+0, 1.127992E-3, 0.000000E+0, 1.276376E+3\r\nE:\\Auswertung_ISS\\data\\011_2018-07-06_17-40-54\\raw_I002_X1_C3.fits.SIM.fits, 8.894713E-1, 1.247808E+0, 1.198987E-3, 0.000000E+0, 1.526828E+3\r\nE:\\Auswertung_ISS\\data\\011_2018-07-06_17-40-54\\raw_I003_X1_C3.fits.SIM.fits, 8.803299E-1, 1.243349E+0, 1.259060E-3, 0.000000E+0, 2.253774E+3\r\nE:\\Auswertung_ISS\\data\\011_2018-07-06_17-40-54\\raw_I004_X1_C3.fits.SIM.fits, 8.729217E-1, 1.221296E+0, 1.258070E-3, 0.000000E+0, 1.315958E+3\r\nE:\\Auswertung_ISS\\data\\011_2018-07-06_17-40-54\\raw_I005_X1_C3.fits.SIM.fits, 8.666606E-1, 1.222119E+0, 1.228481E-3, 0.000000E+0, 1.601187E+3\r\nE:\\Auswertung_ISS\\data\\011_2018-07-06_17-40-54\\raw_I006_X1_C3.fits.SIM.fits, 8.617715E-1, 1.207638E+0, 1.222903E-3, 0.000000E+0, 1.112696E+3\r\nE:\\Auswertung_ISS\\data\\011_2018-07-06_17-40-54\\raw_I007_X1_C3.fits.SIM.fits, 8.575019E-1, 1.199213E+0, 1.294149E-3, 0.000000E+0, 1.241799E+3\r\nE:\\Auswertung_ISS\\data\\011_2018-07-06_17-40-54\\raw_I008_X1_C3.fits.SIM.fits, 8.528828E-1, 1.189822E+0, 1.243138E-3, 0.000000E+0, 1.397659E+3\r\nE:\\Auswertung_ISS\\data\\012_2018-07-07_01-02-54\\raw_I000_X0_C0.fits.SIM.fits, 1.119140E+0, 2.182191E+0, 6.848371E-3, 0.000000E+0, 4.749662E+2\r\nE:\\Auswertung_ISS\\data\\012_2018-07-07_01-02-54\\raw_I000_X0_C1.fits.SIM.fits, 4.259380E+0, 8.789668E+0, 5.592994E-2, 0.000000E+0, 1.255623E+3\r\nE:\\Auswertung_ISS\\data\\012_2018-07-07_01-02-54\\raw_I000_X0_C3.fits.SIM.fits, 2.748620E+0, 4.759268E+0, 6.383035E-3, 0.000000E+0, 1.016953E+3\r\nE:\\Auswertung_ISS\\data\\012_2018-07-07_01-02-54\\raw_I000_X1_C3.fits.SIM.fits, 8.513572E-1, 1.230523E+0, -3.083797E-4, 0.000000E+0, 1.305961E+3\r\nE:\\Auswertung_ISS\\data\\012_2018-07-07_01-02-54\\raw_I001_X1_C3.fits.SIM.fits, 8.369198E-1, 1.200765E+0, 5.996596E-5, 0.000000E+0, 2.188407E+3\r\nE:\\Auswertung_ISS\\data\\012_2018-07-07_01-02-54\\raw_I002_X1_C3.fits.SIM.fits, 8.236085E-1, 1.168511E+0, 1.704766E-4, 0.000000E+0, 1.555732E+3\r\nE:\\Auswertung_ISS\\data\\012_2018-07-07_01-02-54\\raw_I003_X1_C3.fits.SIM.fits, 8.177259E-1, 1.159512E+0, 2.522816E-4, 0.000000E+0, 1.247546E+3\r\nE:\\Auswertung_ISS\\data\\012_2018-07-07_01-02-54\\raw_I004_X1_C3.fits.SIM.fits, 8.107117E-1, 1.147073E+0, 4.044802E-4, 0.000000E+0, 1.017601E+3\r\nE:\\Auswertung_ISS\\data\\012_2018-07-07_01-02-54\\raw_I005_X1_C3.fits.SIM.fits, 8.022652E-1, 1.143616E+0, 4.975566E-4, 0.000000E+0, 1.312425E+3\r\nE:\\Auswertung_ISS\\data\\012_2018-07-07_01-02-54\\raw_I006_X1_C3.fits.SIM.fits, 7.935670E-1, 1.129180E+0, 5.067680E-4, 0.000000E+0, 1.660345E+3\r\nE:\\Auswertung_ISS\\data\\013_2018-07-07_08-02-53\\raw_I000_X0_C0.fits.SIM.fits, 9.614370E-1, 1.895084E+0, 5.175769E-3, 0.000000E+0, 5.623578E+2\r\nE:\\Auswertung_ISS\\data\\013_2018-07-07_08-02-53\\raw_I000_X0_C1.fits.SIM.fits, 3.479417E+0, 8.130126E+0, 4.175507E-2, 0.000000E+0, 1.831009E+3\r\nE:\\Auswertung_ISS\\data\\013_2018-07-07_08-02-53\\raw_I000_X0_C3.fits.SIM.fits, 2.180267E+0, 4.144514E+0, 4.686899E-3, 0.000000E+0, 7.335446E+2\r\nE:\\Auswertung_ISS\\data\\013_2018-07-07_08-02-53\\raw_I000_X1_C0.fits.SIM.fits, 1.511864E+0, 2.187929E+0, -1.135719E-2, 0.000000E+0, 9.395374E+2\r\nE:\\Auswertung_ISS\\data\\013_2018-07-07_08-02-53\\raw_I000_X1_C3.fits.SIM.fits, 9.044187E-1, 1.266304E+0, 1.757874E-3, 0.000000E+0, 9.841819E+2\r\nE:\\Auswertung_ISS\\data\\013_2018-07-07_08-02-53\\raw_I001_X1_C0.fits.SIM.fits, 1.462781E+0, 2.146388E+0, -8.977086E-3, 0.000000E+0, 9.966192E+2\r\nE:\\Auswertung_ISS\\data\\013_2018-07-07_08-02-53\\raw_I001_X1_C3.fits.SIM.fits, 9.013855E-1, 1.268147E+0, 1.915167E-3, 0.000000E+0, 1.256344E+3\r\nE:\\Auswertung_ISS\\data\\013_2018-07-07_08-02-53\\raw_I002_X1_C0.fits.SIM.fits, 1.440405E+0, 2.108274E+0, -8.183194E-3, 0.000000E+0, 1.840396E+3\r\nE:\\Auswertung_ISS\\data\\013_2018-07-07_08-02-53\\raw_I002_X1_C3.fits.SIM.fits, 8.951904E-1, 1.243130E+0, 1.870555E-3, 0.000000E+0, 7.640560E+2\r\nE:\\Auswertung_ISS\\data\\013_2018-07-07_08-02-53\\raw_I003_X1_C0.fits.SIM.fits, 1.421937E+0, 2.065357E+0, -8.030930E-3, 0.000000E+0, 1.436841E+3\r\nE:\\Auswertung_ISS\\data\\013_2018-07-07_08-02-53\\raw_I003_X1_C3.fits.SIM.fits, 8.883269E-1, 1.236043E+0, 1.781967E-3, 0.000000E+0, 1.131214E+3\r\nE:\\Auswertung_ISS\\data\\013_2018-07-07_08-02-53\\raw_I004_X1_C0.fits.SIM.fits, 1.412987E+0, 2.045213E+0, -8.013668E-3, 0.000000E+0, 9.510616E+2\r\nE:\\Auswertung_ISS\\data\\013_2018-07-07_08-02-53\\raw_I004_X1_C3.fits.SIM.fits, 8.837400E-1, 1.225142E+0, 1.840002E-3, 0.000000E+0, 1.017065E+3\r\nE:\\Auswertung_ISS\\data\\013_2018-07-07_08-02-53\\raw_I005_X1_C0.fits.SIM.fits, 1.406077E+0, 2.033173E+0, -7.407173E-3, 0.000000E+0, 7.173264E+2\r\nE:\\Auswertung_ISS\\data\\013_2018-07-07_08-02-53\\raw_I005_X1_C3.fits.SIM.fits, 8.810217E-1, 1.223647E+0, 1.969821E-3, 0.000000E+0, 1.159008E+3\r\nE:\\Auswertung_ISS\\data\\013_2018-07-07_08-02-53\\raw_I006_X1_C0.fits.SIM.fits, 1.400343E+0, 2.022551E+0, -7.557187E-3, 0.000000E+0, 1.485286E+3\r\nE:\\Auswertung_ISS\\data\\013_2018-07-07_08-02-53\\raw_I006_X1_C3.fits.SIM.fits, 8.773603E-1, 1.226421E+0, 1.951632E-3, 0.000000E+0, 1.363987E+3\r\nE:\\Auswertung_ISS\\data\\013_2018-07-07_08-02-53\\raw_I007_X1_C0.fits.SIM.fits, 1.389426E+0, 1.981363E+0, -7.812058E-3, 0.000000E+0, 1.247520E+3\r\nE:\\Auswertung_ISS\\data\\013_2018-07-07_08-02-53\\raw_I007_X1_C3.fits.SIM.fits, 8.738690E-1, 1.209217E+0, 2.190507E-3, 0.000000E+0, 9.259795E+2\r\nE:\\Auswertung_ISS\\data\\013_2018-07-07_08-02-53\\raw_I008_X1_C0.fits.SIM.fits, 1.385072E+0, 1.970862E+0, -7.765111E-3, 0.000000E+0, 8.217391E+2\r\nE:\\Auswertung_ISS\\data\\013_2018-07-07_08-02-53\\raw_I008_X1_C3.fits.SIM.fits, 8.700957E-1, 1.203603E+0, 2.173317E-3, 0.000000E+0, 9.644592E+2\r\nE:\\Auswertung_ISS\\data\\013_2018-07-07_08-02-53\\raw_I009_X1_C0.fits.SIM.fits, 1.387151E+0, 1.994950E+0, -7.037299E-3, 0.000000E+0, 1.008966E+3\r\nE:\\Auswertung_ISS\\data\\013_2018-07-07_08-02-53\\raw_I009_X1_C3.fits.SIM.fits, 8.692407E-1, 1.207454E+0, 2.017877E-3, 0.000000E+0, 1.645209E+3\r\nE:\\Auswertung_ISS\\data\\013_2018-07-07_08-02-53\\raw_I010_X1_C0.fits.SIM.fits, 1.376126E+0, 1.962893E+0, -7.174663E-3, 0.000000E+0, 1.417954E+3\r\nE:\\Auswertung_ISS\\data\\013_2018-07-07_08-02-53\\raw_I010_X1_C3.fits.SIM.fits, 8.668777E-1, 1.201811E+0, 2.075010E-3, 0.000000E+0, 1.075815E+3\r\nE:\\Auswertung_ISS\\data\\013_2018-07-07_08-02-53\\raw_I011_X1_C0.fits.SIM.fits, 1.381089E+0, 1.985917E+0, -6.894142E-3, 0.000000E+0, 1.042353E+3\r\nE:\\Auswertung_ISS\\data\\013_2018-07-07_08-02-53\\raw_I011_X1_C3.fits.SIM.fits, 8.655718E-1, 1.204310E+0, 2.071890E-3, 0.000000E+0, 1.540113E+3\r\nE:\\Auswertung_ISS\\data\\013_2018-07-07_08-02-53\\raw_I012_X1_C0.fits.SIM.fits, 1.377965E+0, 1.977473E+0, -6.811223E-3, 0.000000E+0, 8.321558E+2\r\nE:\\Auswertung_ISS\\data\\013_2018-07-07_08-02-53\\raw_I012_X1_C3.fits.SIM.fits, 8.641844E-1, 1.210382E+0, 2.224003E-3, 0.000000E+0, 1.607130E+3\r\nE:\\Auswertung_ISS\\data\\013_2018-07-07_08-02-53\\raw_I013_X1_C0.fits.SIM.fits, 1.370294E+0, 1.963204E+0, -6.837218E-3, 0.000000E+0, 1.398047E+3\r\nE:\\Auswertung_ISS\\data\\013_2018-07-07_08-02-53\\raw_I013_X1_C3.fits.SIM.fits, 8.636483E-1, 1.195351E+0, 2.041354E-3, 0.000000E+0, 1.361351E+3\r\nE:\\Auswertung_ISS\\data\\013_2018-07-07_08-02-53\\raw_I014_X1_C0.fits.SIM.fits, 1.369378E+0, 1.963905E+0, -6.728539E-3, 0.000000E+0, 1.387452E+3\r\nE:\\Auswertung_ISS\\data\\013_2018-07-07_08-02-53\\raw_I014_X1_C3.fits.SIM.fits, 8.619913E-1, 1.204521E+0, 1.970680E-3, 0.000000E+0, 1.297051E+3\r\nE:\\Auswertung_ISS\\data\\013_2018-07-07_08-02-53\\raw_I015_X1_C0.fits.SIM.fits, 1.363984E+0, 1.935474E+0, -6.987739E-3, 0.000000E+0, 6.912182E+2\r\nE:\\Auswertung_ISS\\data\\013_2018-07-07_08-02-53\\raw_I015_X1_C3.fits.SIM.fits, 8.618423E-1, 1.201349E+0, 2.090285E-3, 0.000000E+0, 1.257311E+3\r\nE:\\Auswertung_ISS\\data\\013_2018-07-07_08-02-53\\raw_I016_X1_C0.fits.SIM.fits, 1.367056E+0, 1.965978E+0, -6.571896E-3, 0.000000E+0, 2.196039E+3\r\nE:\\Auswertung_ISS\\data\\013_2018-07-07_08-02-53\\raw_I016_X1_C3.fits.SIM.fits, 8.619317E-1, 1.200436E+0, 1.925863E-3, 0.000000E+0, 1.590313E+3\r\nE:\\Auswertung_ISS\\data\\013_2018-07-07_08-02-53\\raw_I017_X1_C0.fits.SIM.fits, 1.416742E+0, 2.023776E+0, -8.962677E-3, 0.000000E+0, 1.295045E+3\r\nE:\\Auswertung_ISS\\data\\013_2018-07-07_08-02-53\\raw_I017_X1_C3.fits.SIM.fits, 8.643428E-1, 1.197384E+0, 2.032193E-3, 0.000000E+0, 1.100211E+3\r\nE:\\Auswertung_ISS\\data\\013_2018-07-07_08-02-53\\raw_I018_X1_C0.fits.SIM.fits, 1.420615E+0, 2.012405E+0, -9.743581E-3, 0.000000E+0, 8.109508E+2\r\nE:\\Auswertung_ISS\\data\\013_2018-07-07_08-02-53\\raw_I018_X1_C3.fits.SIM.fits, 8.642746E-1, 1.201224E+0, 1.974007E-3, 0.000000E+0, 1.203353E+3\r\nE:\\Auswertung_ISS\\data\\013_2018-07-07_08-02-53\\raw_I019_X1_C0.fits.SIM.fits, 1.428836E+0, 2.024733E+0, -9.263245E-3, 0.000000E+0, 8.645616E+2\r\nE:\\Auswertung_ISS\\data\\013_2018-07-07_08-02-53\\raw_I019_X1_C3.fits.SIM.fits, 8.691171E-1, 1.205589E+0, 2.130463E-3, 0.000000E+0, 1.138814E+3\r\nE:\\Auswertung_ISS\\data\\013_2018-07-07_08-02-53\\raw_I020_X1_C0.fits.SIM.fits, 1.422274E+0, 2.019560E+0, -9.482816E-3, 0.000000E+0, 1.963371E+3\r\nE:\\Auswertung_ISS\\data\\013_2018-07-07_08-02-53\\raw_I020_X1_C3.fits.SIM.fits, 8.665976E-1, 1.204784E+0, 2.143097E-3, 0.000000E+0, 8.785902E+2\r\nE:\\Auswertung_ISS\\data\\013_2018-07-07_08-02-53\\raw_I021_X1_C0.fits.SIM.fits, 1.416949E+0, 2.002818E+0, -9.693271E-3, 0.000000E+0, 1.187004E+3\r\nE:\\Auswertung_ISS\\data\\013_2018-07-07_08-02-53\\raw_I021_X1_C3.fits.SIM.fits, 8.638883E-1, 1.202266E+0, 1.700220E-3, 0.000000E+0, 9.773237E+2\r\nE:\\Auswertung_ISS\\data\\013_2018-07-07_08-02-53\\raw_I022_X1_C0.fits.SIM.fits, 1.419848E+0, 2.003965E+0, -9.428652E-3, 0.000000E+0, 1.002333E+3\r\nE:\\Auswertung_ISS\\data\\013_2018-07-07_08-02-53\\raw_I022_X1_C3.fits.SIM.fits, 8.636153E-1, 1.199266E+0, 1.741063E-3, 0.000000E+0, 1.120612E+3\r\nE:\\Auswertung_ISS\\data\\013_2018-07-07_08-02-53\\raw_I023_X1_C0.fits.SIM.fits, 1.428040E+0, 2.014615E+0, -9.292263E-3, 0.000000E+0, 1.035895E+3\r\nE:\\Auswertung_ISS\\data\\013_2018-07-07_08-02-53\\raw_I023_X1_C3.fits.SIM.fits, 8.718544E-1, 1.210120E+0, 1.851314E-3, 0.000000E+0, 1.236908E+3\r\nE:\\Auswertung_ISS\\data\\013_2018-07-07_08-02-53\\raw_I024_X1_C0.fits.SIM.fits, 1.424462E+0, 2.007619E+0, -9.338942E-3, 0.000000E+0, 1.103425E+3\r\nE:\\Auswertung_ISS\\data\\013_2018-07-07_08-02-53\\raw_I024_X1_C3.fits.SIM.fits, 8.681094E-1, 1.209510E+0, 1.882254E-3, 0.000000E+0, 1.381801E+3\r\nE:\\Auswertung_ISS\\data\\013_2018-07-07_08-02-53\\raw_I025_X1_C0.fits.SIM.fits, 1.424180E+0, 2.003645E+0, -9.381469E-3, 0.000000E+0, 8.691588E+2\r\nE:\\Auswertung_ISS\\data\\013_2018-07-07_08-02-53\\raw_I025_X1_C3.fits.SIM.fits, 8.756796E-1, 1.227607E+0, 1.546950E-3, 0.000000E+0, 1.632576E+3\r\nE:\\Auswertung_ISS\\data\\013_2018-07-07_08-02-53\\raw_I026_X1_C0.fits.SIM.fits, 1.417791E+0, 1.995619E+0, -9.400791E-3, 0.000000E+0, 9.183976E+2\r\nE:\\Auswertung_ISS\\data\\013_2018-07-07_08-02-53\\raw_I026_X1_C3.fits.SIM.fits, 8.717192E-1, 1.214511E+0, 1.611517E-3, 0.000000E+0, 1.247270E+3\r\nE:\\Auswertung_ISS\\data\\013_2018-07-07_08-02-53\\raw_I027_X1_C0.fits.SIM.fits, 1.431988E+0, 2.015526E+0, -9.127689E-3, 0.000000E+0, 1.309282E+3\r\nE:\\Auswertung_ISS\\data\\013_2018-07-07_08-02-53\\raw_I027_X1_C3.fits.SIM.fits, 8.793476E-1, 1.223806E+0, 1.966172E-3, 0.000000E+0, 1.058300E+3\r\nE:\\Auswertung_ISS\\data\\013_2018-07-07_08-02-53\\raw_I028_X1_C0.fits.SIM.fits, 1.429031E+0, 2.007186E+0, -8.936664E-3, 0.000000E+0, 9.230627E+2\r\nE:\\Auswertung_ISS\\data\\013_2018-07-07_08-02-53\\raw_I028_X1_C3.fits.SIM.fits, 8.787970E-1, 1.221269E+0, 1.746475E-3, 0.000000E+0, 1.231505E+3\r\nE:\\Auswertung_ISS\\data\\013_2018-07-07_08-02-53\\raw_I029_X1_C0.fits.SIM.fits, 1.425592E+0, 2.002615E+0, -9.145387E-3, 0.000000E+0, 1.319157E+3\r\nE:\\Auswertung_ISS\\data\\013_2018-07-07_08-02-53\\raw_I029_X1_C3.fits.SIM.fits, 8.753410E-1, 1.228053E+0, 1.645251E-3, 0.000000E+0, 1.342796E+3\r\nE:\\Auswertung_ISS\\data\\014_2018-07-16_17-53-52\\raw_I000_X0_C0.fits.SIM.fits, 9.529770E-1, 1.935869E+0, 6.138332E-3, 0.000000E+0, 7.344355E+2\r\nE:\\Auswertung_ISS\\data\\014_2018-07-16_17-53-52\\raw_I000_X0_C1.fits.SIM.fits, 3.389503E+0, 7.901408E+0, 3.951946E-2, 0.000000E+0, 1.758199E+3\r\nE:\\Auswertung_ISS\\data\\014_2018-07-16_17-53-52\\raw_I000_X0_C3.fits.SIM.fits, 1.087207E+0, 1.800494E+0, 2.239728E-3, 0.000000E+0, 3.376852E+2\r\nE:\\Auswertung_ISS\\data\\014_2018-07-16_17-53-52\\raw_I000_X1_C0.fits.SIM.fits, 1.448817E+0, 2.031656E+0, -9.723802E-3, 0.000000E+0, 2.555999E+3\r\nE:\\Auswertung_ISS\\data\\014_2018-07-16_17-53-52\\raw_I000_X1_C3.fits.SIM.fits, 8.753798E-1, 1.231656E+0, 1.564622E-3, 0.000000E+0, 1.296684E+3\r\nE:\\Auswertung_ISS\\data\\014_2018-07-16_17-53-52\\raw_I001_X1_C0.fits.SIM.fits, 1.407988E+0, 1.971809E+0, -7.260683E-3, 0.000000E+0, 1.369470E+3\r\nE:\\Auswertung_ISS\\data\\014_2018-07-16_17-53-52\\raw_I001_X1_C3.fits.SIM.fits, 8.672975E-1, 1.227324E+0, 1.101702E-3, 0.000000E+0, 1.291759E+3\r\nE:\\Auswertung_ISS\\data\\014_2018-07-16_17-53-52\\raw_I002_X1_C0.fits.SIM.fits, 1.396450E+0, 1.951073E+0, -6.898039E-3, 0.000000E+0, 9.740944E+2\r\nE:\\Auswertung_ISS\\data\\014_2018-07-16_17-53-52\\raw_I002_X1_C3.fits.SIM.fits, 8.639990E-1, 1.214733E+0, 1.176298E-3, 0.000000E+0, 1.450438E+3\r\nE:\\Auswertung_ISS\\data\\014_2018-07-16_17-53-52\\raw_I003_X1_C0.fits.SIM.fits, 1.389792E+0, 1.942054E+0, -6.417855E-3, 0.000000E+0, 9.621342E+2\r\nE:\\Auswertung_ISS\\data\\014_2018-07-16_17-53-52\\raw_I003_X1_C3.fits.SIM.fits, 8.656155E-1, 1.217611E+0, 1.110294E-3, 0.000000E+0, 1.468672E+3\r\nE:\\Auswertung_ISS\\data\\014_2018-07-16_17-53-52\\raw_I004_X1_C0.fits.SIM.fits, 1.386367E+0, 1.942419E+0, -6.006109E-3, 0.000000E+0, 1.255411E+3\r\nE:\\Auswertung_ISS\\data\\014_2018-07-16_17-53-52\\raw_I004_X1_C3.fits.SIM.fits, 8.654237E-1, 1.216759E+0, 1.020892E-3, 0.000000E+0, 9.332996E+2\r\nE:\\Auswertung_ISS\\data\\014_2018-07-16_17-53-52\\raw_I005_X1_C0.fits.SIM.fits, 1.381190E+0, 1.931680E+0, -5.886421E-3, 0.000000E+0, 6.721239E+2\r\nE:\\Auswertung_ISS\\data\\014_2018-07-16_17-53-52\\raw_I005_X1_C3.fits.SIM.fits, 8.654640E-1, 1.215075E+0, 8.619290E-4, 0.000000E+0, 1.401830E+3\r\nE:\\Auswertung_ISS\\data\\014_2018-07-16_17-53-52\\raw_I006_X1_C0.fits.SIM.fits, 1.379361E+0, 1.927269E+0, -5.720602E-3, 0.000000E+0, 8.988006E+2\r\nE:\\Auswertung_ISS\\data\\014_2018-07-16_17-53-52\\raw_I006_X1_C3.fits.SIM.fits, 8.657628E-1, 1.216832E+0, 1.049576E-3, 0.000000E+0, 9.196039E+2\r\nE:\\Auswertung_ISS\\data\\014_2018-07-16_17-53-52\\raw_I007_X1_C0.fits.SIM.fits, 1.375879E+0, 1.927058E+0, -5.417695E-3, 0.000000E+0, 9.542994E+2\r\nE:\\Auswertung_ISS\\data\\014_2018-07-16_17-53-52\\raw_I007_X1_C3.fits.SIM.fits, 8.639175E-1, 1.212562E+0, 8.735683E-4, 0.000000E+0, 1.186842E+3\r\nE:\\Auswertung_ISS\\data\\014_2018-07-16_17-53-52\\raw_I008_X1_C0.fits.SIM.fits, 1.376049E+0, 1.925494E+0, -5.546401E-3, 0.000000E+0, 9.946210E+2\r\nE:\\Auswertung_ISS\\data\\014_2018-07-16_17-53-52\\raw_I008_X1_C3.fits.SIM.fits, 8.653361E-1, 1.211768E+0, 8.540409E-4, 0.000000E+0, 1.052115E+3\r\nE:\\Auswertung_ISS\\data\\014_2018-07-16_17-53-52\\raw_I009_X1_C0.fits.SIM.fits, 1.372908E+0, 1.924158E+0, -5.383443E-3, 0.000000E+0, 1.148381E+3\r\nE:\\Auswertung_ISS\\data\\014_2018-07-16_17-53-52\\raw_I009_X1_C3.fits.SIM.fits, 8.660708E-1, 1.211440E+0, 9.560139E-4, 0.000000E+0, 1.287434E+3\r\nE:\\Auswertung_ISS\\data\\014_2018-07-16_17-53-52\\raw_I010_X1_C0.fits.SIM.fits, 1.369534E+0, 1.921370E+0, -5.153595E-3, 0.000000E+0, 1.158746E+3\r\nE:\\Auswertung_ISS\\data\\014_2018-07-16_17-53-52\\raw_I010_X1_C3.fits.SIM.fits, 8.640471E-1, 1.218946E+0, 7.441225E-4, 0.000000E+0, 1.270107E+3\r\nE:\\Auswertung_ISS\\data\\014_2018-07-16_17-53-52\\raw_I011_X1_C0.fits.SIM.fits, 1.367456E+0, 1.924945E+0, -4.962616E-3, 0.000000E+0, 1.542481E+3\r\nE:\\Auswertung_ISS\\data\\014_2018-07-16_17-53-52\\raw_I011_X1_C3.fits.SIM.fits, 8.636880E-1, 1.219360E+0, 8.809239E-4, 0.000000E+0, 1.051712E+3\r\nE:\\Auswertung_ISS\\data\\014_2018-07-16_17-53-52\\raw_I012_X1_C0.fits.SIM.fits, 1.366812E+0, 1.917810E+0, -4.840869E-3, 0.000000E+0, 9.042333E+2\r\nE:\\Auswertung_ISS\\data\\014_2018-07-16_17-53-52\\raw_I012_X1_C3.fits.SIM.fits, 8.643230E-1, 1.222740E+0, 8.305277E-4, 0.000000E+0, 1.894740E+3\r\nE:\\Auswertung_ISS\\data\\014_2018-07-16_17-53-52\\raw_I013_X1_C0.fits.SIM.fits, 1.367576E+0, 1.918543E+0, -4.723137E-3, 0.000000E+0, 1.188615E+3\r\nE:\\Auswertung_ISS\\data\\014_2018-07-16_17-53-52\\raw_I013_X1_C3.fits.SIM.fits, 8.646900E-1, 1.210917E+0, 7.735836E-4, 0.000000E+0, 8.842684E+2\r\nE:\\Auswertung_ISS\\data\\014_2018-07-16_17-53-52\\raw_I014_X1_C0.fits.SIM.fits, 1.366196E+0, 1.913505E+0, -4.823416E-3, 0.000000E+0, 1.096467E+3\r\nE:\\Auswertung_ISS\\data\\014_2018-07-16_17-53-52\\raw_I014_X1_C3.fits.SIM.fits, 8.638858E-1, 1.221548E+0, 7.942717E-4, 0.000000E+0, 1.710234E+3\r\nE:\\Auswertung_ISS\\data\\014_2018-07-16_17-53-52\\raw_I015_X1_C0.fits.SIM.fits, 1.365989E+0, 1.913512E+0, -4.618713E-3, 0.000000E+0, 8.493683E+2\r\nE:\\Auswertung_ISS\\data\\014_2018-07-16_17-53-52\\raw_I015_X1_C3.fits.SIM.fits, 8.645261E-1, 1.226739E+0, 9.600011E-4, 0.000000E+0, 1.479982E+3\r\nE:\\Auswertung_ISS\\data\\014_2018-07-16_17-53-52\\raw_I016_X1_C0.fits.SIM.fits, 1.368812E+0, 1.917382E+0, -4.392201E-3, 0.000000E+0, 1.085804E+3\r\nE:\\Auswertung_ISS\\data\\014_2018-07-16_17-53-52\\raw_I016_X1_C3.fits.SIM.fits, 8.662847E-1, 1.218020E+0, 1.036865E-3, 0.000000E+0, 1.226787E+3\r\nE:\\Auswertung_ISS\\data\\014_2018-07-16_17-53-52\\raw_I017_X1_C0.fits.SIM.fits, 1.400522E+0, 1.952782E+0, -6.054147E-3, 0.000000E+0, 8.819812E+2\r\nE:\\Auswertung_ISS\\data\\014_2018-07-16_17-53-52\\raw_I017_X1_C3.fits.SIM.fits, 8.768019E-1, 1.231897E+0, 1.253598E-3, 0.000000E+0, 1.476238E+3\r\nE:\\Auswertung_ISS\\data\\014_2018-07-16_17-53-52\\raw_I018_X1_C0.fits.SIM.fits, 1.403182E+0, 1.961734E+0, -6.151350E-3, 0.000000E+0, 1.411117E+3\r\nE:\\Auswertung_ISS\\data\\014_2018-07-16_17-53-52\\raw_I018_X1_C3.fits.SIM.fits, 8.751565E-1, 1.238297E+0, 1.144850E-3, 0.000000E+0, 1.275655E+3\r\nE:\\Auswertung_ISS\\data\\014_2018-07-16_17-53-52\\raw_I019_X1_C0.fits.SIM.fits, 1.400845E+0, 1.953452E+0, -6.245568E-3, 0.000000E+0, 8.696378E+2\r\nE:\\Auswertung_ISS\\data\\014_2018-07-16_17-53-52\\raw_I019_X1_C3.fits.SIM.fits, 8.710193E-1, 1.232547E+0, 1.036724E-3, 0.000000E+0, 1.087018E+3\r\nE:\\Auswertung_ISS\\data\\014_2018-07-16_17-53-52\\raw_I020_X1_C0.fits.SIM.fits, 1.401899E+0, 1.955364E+0, -5.921845E-3, 0.000000E+0, 8.892388E+2\r\nE:\\Auswertung_ISS\\data\\014_2018-07-16_17-53-52\\raw_I020_X1_C3.fits.SIM.fits, 8.694855E-1, 1.230708E+0, 7.241330E-4, 0.000000E+0, 1.323332E+3\r\nE:\\Auswertung_ISS\\data\\014_2018-07-16_17-53-52\\raw_I021_X1_C0.fits.SIM.fits, 1.401820E+0, 1.953420E+0, -5.707627E-3, 0.000000E+0, 7.153414E+2\r\nE:\\Auswertung_ISS\\data\\014_2018-07-16_17-53-52\\raw_I021_X1_C3.fits.SIM.fits, 8.691770E-1, 1.217774E+0, 9.941545E-4, 0.000000E+0, 1.157790E+3\r\nE:\\Auswertung_ISS\\data\\014_2018-07-16_17-53-52\\raw_I022_X1_C0.fits.SIM.fits, 1.401918E+0, 1.957982E+0, -5.809768E-3, 0.000000E+0, 1.179954E+3\r\nE:\\Auswertung_ISS\\data\\014_2018-07-16_17-53-52\\raw_I022_X1_C3.fits.SIM.fits, 8.647231E-1, 1.215170E+0, 8.804640E-4, 0.000000E+0, 1.081741E+3\r\nE:\\Auswertung_ISS\\data\\014_2018-07-16_17-53-52\\raw_I023_X1_C0.fits.SIM.fits, 1.396599E+0, 1.949613E+0, -5.564629E-3, 0.000000E+0, 1.272092E+3\r\nE:\\Auswertung_ISS\\data\\014_2018-07-16_17-53-52\\raw_I023_X1_C3.fits.SIM.fits, 8.618402E-1, 1.220440E+0, 8.032709E-4, 0.000000E+0, 1.600411E+3\r\nE:\\Auswertung_ISS\\data\\014_2018-07-16_17-53-52\\raw_I024_X1_C0.fits.SIM.fits, 1.398839E+0, 1.953949E+0, -5.305773E-3, 0.000000E+0, 1.215996E+3\r\nE:\\Auswertung_ISS\\data\\014_2018-07-16_17-53-52\\raw_I024_X1_C3.fits.SIM.fits, 8.612819E-1, 1.216403E+0, 7.470950E-4, 0.000000E+0, 1.207291E+3\r\nE:\\Auswertung_ISS\\data\\014_2018-07-16_17-53-52\\raw_I025_X1_C0.fits.SIM.fits, 1.399332E+0, 1.949334E+0, -5.061780E-3, 0.000000E+0, 9.511170E+2\r\nE:\\Auswertung_ISS\\data\\014_2018-07-16_17-53-52\\raw_I025_X1_C3.fits.SIM.fits, 8.590943E-1, 1.201704E+0, 6.738738E-4, 0.000000E+0, 1.020165E+3\r\nE:\\Auswertung_ISS\\data\\014_2018-07-16_17-53-52\\raw_I026_X1_C0.fits.SIM.fits, 1.406048E+0, 1.959883E+0, -4.518550E-3, 0.000000E+0, 8.163887E+2\r\nE:\\Auswertung_ISS\\data\\014_2018-07-16_17-53-52\\raw_I026_X1_C3.fits.SIM.fits, 8.610812E-1, 1.208851E+0, 8.459689E-4, 0.000000E+0, 1.196879E+3\r\nE:\\Auswertung_ISS\\data\\014_2018-07-16_17-53-52\\raw_I027_X1_C0.fits.SIM.fits, 1.401200E+0, 1.955720E+0, -4.453071E-3, 0.000000E+0, 1.074010E+3\r\nE:\\Auswertung_ISS\\data\\014_2018-07-16_17-53-52\\raw_I027_X1_C3.fits.SIM.fits, 8.561412E-1, 1.197752E+0, 5.380258E-4, 0.000000E+0, 1.118977E+3\r\nE:\\Auswertung_ISS\\data\\014_2018-07-16_17-53-52\\raw_I028_X1_C0.fits.SIM.fits, 1.403272E+0, 1.955919E+0, -4.055736E-3, 0.000000E+0, 9.104365E+2\r\nE:\\Auswertung_ISS\\data\\014_2018-07-16_17-53-52\\raw_I028_X1_C3.fits.SIM.fits, 8.554013E-1, 1.192764E+0, 8.834581E-4, 0.000000E+0, 1.144379E+3\r\nE:\\Auswertung_ISS\\data\\014_2018-07-16_17-53-52\\raw_I029_X1_C0.fits.SIM.fits, 1.403855E+0, 1.956581E+0, -3.487078E-3, 0.000000E+0, 1.462673E+3\r\nE:\\Auswertung_ISS\\data\\014_2018-07-16_17-53-52\\raw_I029_X1_C3.fits.SIM.fits, 8.562182E-1, 1.203721E+0, 1.004740E-3, 0.000000E+0, 1.211450E+3\r\n"
  out "working":i32=366
  in  "All Files in Dir":path[](array[path])=[path "E:/Auswertung_ISS/data/002_2018-06-21_16-44-14/raw_I000_X0_C0.fits.SIM.fits", path "E:/Auswertung_ISS/data/002_2018-06-21_16-44-14/raw_I000_X0_C1.fits.SIM.fits", path "E:/Auswertung_ISS/data/002_2018-06-21_16-44-14/raw_I000_X0_C3.fits.SIM.fits", path "E:/Auswertung_ISS/data/002_2018-06-21_16-44-14/raw_I000_X1_C0.fits.SIM.fits", path "E:/Auswertung_ISS/data/002_2018-06-21_16-44-14/raw_I000_X1_C3.fits.SIM.fits", path "E:/Auswertung_ISS/data/003_2018-07-03_15-08-29/raw_I000_X0_C0.fits.SIM.fits", path "E:/Auswertung_ISS/data/003_2018-07-03_15-08-29/raw_I000_X0_C1.fits.SIM.fits", path "E:/Auswertung_ISS/data/003_2018-07-03_15-08-29/raw_I000_X0_C3.fits.SIM.fits", path "E:/Auswertung_ISS/data/003_2018-07-03_15-08-29/raw_I000_X1_C0.fits.SIM.fits", path "E:/Auswertung_ISS/data/003_2018-07-03_15-08-29/raw_I000_X1_C3.fits.SIM.fits", path "E:/Auswertung_ISS/data/003_2018-07-03_15-08-29/raw_I001_X1_C0.fits.SIM.fits", path "E:/Auswertung_ISS/data/003_2018-07-03_15-08-29/raw_I001_X1_C3.fits.SIM.fits", path "E:/Auswertung_ISS/data/003_2018-07-03_15-08-29/raw_I002_X1_C0.fits.SIM.fits", path "E:/Auswertung_ISS/data/003_2018-07-03_15-08-29/raw_I002_X1_C3.fits.SIM.fits", path "E:/Auswertung_ISS/data/003_2018-07-03_15-08-29/raw_I003_X1_C0.fits.SIM.fits", path "E:/Auswertung_ISS/data/003_2018-07-03_15-08-29/raw_I003_X1_C3.fits.SIM.fits", path "E:/Auswertung_ISS/data/003_2018-07-03_15-08-29/raw_I004_X1_C0.fits.SIM.fits", path "E:/Auswertung_ISS/data/003_2018-07-03_15-08-29/raw_I004_X1_C3.fits.SIM.fits", path "E:/Auswertung_ISS/data/003_2018-07-03_15-08-29/raw_I005_X1_C0.fits.SIM.fits", path "E:/Auswertung_ISS/data/003_2018-07-03_15-08-29/raw_I005_X1_C3.fits.SIM.fits", path "E:/Auswertung_ISS/data/003_2018-07-03_15-08-29/raw_I006_X1_C0.fits.SIM.fits", path "E:/Auswertung_ISS/data/003_2018-07-03_15-08-29/raw_I006_X1_C3.fits.SIM.fits", path "E:/Auswertung_ISS/data/003_2018-07-03_15-08-29/raw_I007_X1_C0.fits.SIM.fits", path "E:/Auswertung_ISS/data/003_2018-07-03_15-08-29/raw_I007_X1_C3.fits.SIM.fits", path "E:/Auswertung_ISS/data/003_2018-07-03_15-08-29/raw_I008_X1_C0.fits.SIM.fits", path "E:/Auswertung_ISS/data/003_2018-07-03_15-08-29/raw_I008_X1_C3.fits.SIM.fits", path "E:/Auswertung_ISS/data/003_2018-07-03_15-08-29/raw_I009_X0_C0.fits.SIM.fits", path "E:/Auswertung_ISS/data/003_2018-07-03_15-08-29/raw_I009_X0_C1.fits.SIM.fits", path "E:/Auswertung_ISS/data/003_2018-07-03_15-08-29/raw_I009_X0_C3.fits.SIM.fits", path "E:/Auswertung_ISS/data/003_2018-07-03_15-08-29/raw_I009_X1_C0.fits.SIM.fits", path "E:/Auswertung_ISS/data/003_2018-07-03_15-08-29/raw_I009_X1_C3.fits.SIM.fits", path "E:/Auswertung_ISS/data/004_2018-07-03_17-33-15/raw_I000_X0_C0.fits.SIM.fits", path "E:/Auswertung_ISS/data/004_2018-07-03_17-33-15/raw_I000_X0_C1.fits.SIM.fits", path "E:/Auswertung_ISS/data/004_2018-07-03_17-33-15/raw_I000_X0_C3.fits.SIM.fits", path "E:/Auswertung_ISS/data/004_2018-07-03_17-33-15/raw_I000_X1_C0.fits.SIM.fits", path "E:/Auswertung_ISS/data/004_2018-07-03_17-33-15/raw_I000_X1_C3.fits.SIM.fits", path "E:/Auswertung_ISS/data/004_2018-07-03_17-33-15/raw_I001_X1_C0.fits.SIM.fits", path "E:/Auswertung_ISS/data/004_2018-07-03_17-33-15/raw_I001_X1_C3.fits.SIM.fits", path "E:/Auswertung_ISS/data/004_2018-07-03_17-33-15/raw_I002_X1_C0.fits.SIM.fits", path "E:/Auswertung_ISS/data/004_2018-07-03_17-33-15/raw_I002_X1_C3.fits.SIM.fits", path "E:/Auswertung_ISS/data/004_2018-07-03_17-33-15/raw_I003_X1_C0.fits.SIM.fits", path "E:/Auswertung_ISS/data/004_2018-07-03_17-33-15/raw_I003_X1_C3.fits.SIM.fits", path "E:/Auswertung_ISS/data/004_2018-07-03_17-33-15/raw_I004_X1_C0.fits.SIM.fits", path "E:/Auswertung_ISS/data/004_2018-07-03_17-33-15/raw_I004_X1_C3.fits.SIM.fits", path "E:/Auswertung_ISS/data/004_2018-07-03_17-33-15/raw_I005_X1_C0.fits.SIM.fits", path "E:/Auswertung_ISS/data/004_2018-07-03_17-33-15/raw_I005_X1_C3.fits.SIM.fits", path "E:/Auswertung_ISS/data/004_2018-07-03_17-33-15/raw_I006_X1_C0.fits.SIM.fits", path "E:/Auswertung_ISS/data/004_2018-07-03_17-33-15/raw_I006_X1_C3.fits.SIM.fits", path "E:/Auswertung_ISS/data/004_2018-07-03_17-33-15/raw_I007_X1_C0.fits.SIM.fits", path "E:/Auswertung_ISS/data/004_2018-07-03_17-33-15/raw_I007_X1_C3.fits.SIM.fits", path "E:/Auswertung_ISS/data/004_2018-07-03_17-33-15/raw_I008_X1_C0.fits.SIM.fits", path "E:/Auswertung_ISS/data/004_2018-07-03_17-33-15/raw_I008_X1_C3.fits.SIM.fits", path "E:/Auswertung_ISS/data/004_2018-07-03_17-33-15/raw_I009_X1_C0.fits.SIM.fits", path "E:/Auswertung_ISS/data/004_2018-07-03_17-33-15/raw_I009_X1_C3.fits.SIM.fits", path "E:/Auswertung_ISS/data/004_2018-07-03_17-33-15/raw_I010_X1_C0.fits.SIM.fits", path "E:/Auswertung_ISS/data/004_2018-07-03_17-33-15/raw_I010_X1_C3.fits.SIM.fits", path "E:/Auswertung_ISS/data/004_2018-07-03_17-33-15/raw_I011_X1_C0.fits.SIM.fits", path "E:/Auswertung_ISS/data/004_2018-07-03_17-33-15/raw_I011_X1_C3.fits.SIM.fits", path "E:/Auswertung_ISS/data/004_2018-07-03_17-33-15/raw_I012_X1_C0.fits.SIM.fits", path "E:/Auswertung_ISS/data/004_2018-07-03_17-33-15/raw_I012_X1_C3.fits.SIM.fits", path "E:/Auswertung_ISS/data/004_2018-07-03_17-33-15/raw_I013_X1_C0.fits.SIM.fits", path "E:/Auswertung_ISS/data/004_2018-07-03_17-33-15/raw_I013_X1_C3.fits.SIM.fits", path "E:/Auswertung_ISS/data/004_2018-07-03_17-33-15/raw_I014_X1_C0.fits.SIM.fits", path "E:/Auswertung_ISS/data/004_2018-07-03_17-33-15/raw_I014_X1_C3.fits.SIM.fits", path "E:/Auswertung_ISS/data/004_2018-07-03_17-33-15/raw_I015_X1_C0.fits.SIM.fits", path "E:/Auswertung_ISS/data/004_2018-07-03_17-33-15/raw_I015_X1_C3.fits.SIM.fits", path "E:/Auswertung_ISS/data/004_2018-07-03_17-33-15/raw_I016_X1_C0.fits.SIM.fits", path "E:/Auswertung_ISS/data/004_2018-07-03_17-33-15/raw_I016_X1_C3.fits.SIM.fits", path "E:/Auswertung_ISS/data/004_2018-07-03_17-33-15/raw_I017_X1_C0.fits.SIM.fits", path "E:/Auswertung_ISS/data/004_2018-07-03_17-33-15/raw_I017_X1_C3.fits.SIM.fits", path "E:/Auswertung_ISS/data/005_2018-07-04_08-02-54/raw_I000_X0_C0.fits.SIM.fits", path "E:/Auswertung_ISS/data/005_2018-07-04_08-02-54/raw_I000_X0_C1.fits.SIM.fits", path "E:/Auswertung_ISS/data/005_2018-07-04_08-02-54/raw_I000_X0_C3.fits.SIM.fits", path "E:/Auswertung_ISS/data/005_2018-07-04_08-02-54/raw_I000_X1_C0.fits.SIM.fits", path "E:/Auswertung_ISS/data/005_2018-07-04_08-02-54/raw_I000_X1_C3.fits.SIM.fits", path "E:/Auswertung_ISS/data/005_2018-07-04_08-02-54/raw_I001_X1_C0.fits.SIM.fits", path "E:/Auswertung_ISS/data/005_2018-07-04_08-02-54/raw_I001_X1_C3.fits.SIM.fits", path "E:/Auswertung_ISS/data/005_2018-07-04_08-02-54/raw_I002_X1_C0.fits.SIM.fits", path "E:/Auswertung_ISS/data/005_2018-07-04_08-02-54/raw_I002_X1_C3.fits.SIM.fits", path "E:/Auswertung_ISS/data/005_2018-07-04_08-02-54/raw_I003_X1_C0.fits.SIM.fits", path "E:/Auswertung_ISS/data/005_2018-07-04_08-02-54/raw_I003_X1_C3.fits.SIM.fits", path "E:/Auswertung_ISS/data/005_2018-07-04_08-02-54/raw_I004_X1_C0.fits.SIM.fits", path "E:/Auswertung_ISS/data/005_2018-07-04_08-02-54/raw_I004_X1_C3.fits.SIM.fits", path "E:/Auswertung_ISS/data/005_2018-07-04_08-02-54/raw_I005_X1_C0.fits.SIM.fits", path "E:/Auswertung_ISS/data/005_2018-07-04_08-02-54/raw_I005_X1_C3.fits.SIM.fits", path "E:/Auswertung_ISS/data/005_2018-07-04_08-02-54/raw_I006_X1_C0.fits.SIM.fits", path "E:/Auswertung_ISS/data/005_2018-07-04_08-02-54/raw_I006_X1_C3.fits.SIM.fits", path "E:/Auswertung_ISS/data/005_2018-07-04_08-02-54/raw_I007_X1_C0.fits.SIM.fits", path "E:/Auswertung_ISS/data/005_2018-07-04_08-02-54/raw_I007_X1_C3.fits.SIM.fits", path "E:/Auswertung_ISS/data/005_2018-07-04_08-02-54/raw_I008_X1_C0.fits.SIM.fits", path "E:/Auswertung_ISS/data/005_2018-07-04_08-02-54/raw_I008_X1_C3.fits.SIM.fits", path "E:/Auswertung_ISS/data/005_2018-07-04_08-02-54/raw_I009_X1_C0.fits.SIM.fits", path "E:/Auswertung_ISS/data/005_2018-07-04_08-02-54/raw_I009_X1_C3.fits.SIM.fits", path "E:/Auswertung_ISS/data/005_2018-07-04_08-02-54/raw_I010_X1_C0.fits.SIM.fits", path "E:/Auswertung_ISS/data/005_2018-07-04_08-02-54/raw_I010_X1_C3.fits.SIM.fits", path "E:/Auswertung_ISS/data/005_2018-07-04_08-02-54/raw_I011_X1_C0.fits.SIM.fits", path "E:/Auswertung_ISS/data/005_2018-07-04_08-02-54/raw_I011_X1_C3.fits.SIM.fits", path "E:/Auswertung_ISS/data/005_2018-07-04_08-02-54/raw_I012_X1_C0.fits.SIM.fits", path "E:/Auswertung_ISS/data/005_2018-07-04_08-02-54/raw_I012_X1_C3.fits.SIM.fits", path "E:/Auswertung_ISS/data/005_2018-07-04_08-02-54/raw_I013_X1_C0.fits.SIM.fits", path "E:/Auswertung_ISS/data/005_2018-07-04_08-02-54/raw_I013_X1_C3.fits.SIM.fits", path "E:/Auswertung_ISS/data/005_2018-07-04_08-02-54/raw_I014_X1_C0.fits.SIM.fits", path "E:/Auswertung_ISS/data/005_2018-07-04_08-02-54/raw_I014_X1_C3.fits.SIM.fits", path "E:/Auswertung_ISS/data/005_2018-07-04_08-02-54/raw_I015_X1_C0.fits.SIM.fits", path "E:/Auswertung_ISS/data/005_2018-07-04_08-02-54/raw_I015_X1_C3.fits.SIM.fits", path "E:/Auswertung_ISS/data/005_2018-07-04_08-02-54/raw_I016_X1_C0.fits.SIM.fits", path "E:/Auswertung_ISS/data/005_2018-07-04_08-02-54/raw_I016_X1_C3.fits.SIM.fits", path "E:/Auswertung_ISS/data/006_2018-07-04_15-43-18/raw_I000_X0_C0.fits.SIM.fits", path "E:/Auswertung_ISS/data/006_2018-07-04_15-43-18/raw_I000_X0_C1.fits.SIM.fits", path "E:/Auswertung_ISS/data/006_2018-07-04_15-43-18/raw_I000_X0_C3.fits.SIM.fits", path "E:/Auswertung_ISS/data/006_2018-07-04_15-43-18/raw_I000_X1_C0.fits.SIM.fits", path "E:/Auswertung_ISS/data/006_2018-07-04_15-43-18/raw_I000_X1_C3.fits.SIM.fits", path "E:/Auswertung_ISS/data/006_2018-07-04_15-43-18/raw_I001_X1_C0.fits.SIM.fits", path "E:/Auswertung_ISS/data/006_2018-07-04_15-43-18/raw_I001_X1_C3.fits.SIM.fits", path "E:/Auswertung_ISS/data/006_2018-07-04_15-43-18/raw_I002_X1_C0.fits.SIM.fits", path "E:/Auswertung_ISS/data/006_2018-07-04_15-43-18/raw_I002_X1_C3.fits.SIM.fits", path "E:/Auswertung_ISS/data/006_2018-07-04_15-43-18/raw_I003_X1_C0.fits.SIM.fits", path "E:/Auswertung_ISS/data/006_2018-07-04_15-43-18/raw_I003_X1_C3.fits.SIM.fits", path "E:/Auswertung_ISS/data/007_2018-07-04_16-44-22/raw_I000_X0_C0.fits.SIM.fits", path "E:/Auswertung_ISS/data/007_2018-07-04_16-44-22/raw_I000_X0_C1.fits.SIM.fits", path "E:/Auswertung_ISS/data/007_2018-07-04_16-44-22/raw_I000_X0_C3.fits.SIM.fits", path "E:/Auswertung_ISS/data/007_2018-07-04_16-44-22/raw_I000_X1_C0.fits.SIM.fits", path "E:/Auswertung_ISS/data/007_2018-07-04_16-44-22/raw_I000_X1_C3.fits.SIM.fits", path "E:/Auswertung_ISS/data/007_2018-07-04_16-44-22/raw_I001_X1_C0.fits.SIM.fits", path "E:/Auswertung_ISS/data/007_2018-07-04_16-44-22/raw_I001_X1_C3.fits.SIM.fits", path "E:/Auswertung_ISS/data/007_2018-07-04_16-44-22/raw_I002_X1_C0.fits.SIM.fits", path "E:/Auswertung_ISS/data/007_2018-07-04_16-44-22/raw_I002_X1_C3.fits.SIM.fits", path "E:/Auswertung_ISS/data/007_2018-07-04_16-44-22/raw_I003_X1_C0.fits.SIM.fits", path "E:/Auswertung_ISS/data/007_2018-07-04_16-44-22/raw_I003_X1_C3.fits.SIM.fits", path "E:/Auswertung_ISS/data/007_2018-07-04_16-44-22/raw_I004_X1_C0.fits.SIM.fits", path "E:/Auswertung_ISS/data/007_2018-07-04_16-44-22/raw_I004_X1_C3.fits.SIM.fits", path "E:/Auswertung_ISS/data/007_2018-07-04_16-44-22/raw_I005_X1_C0.fits.SIM.fits", path "E:/Auswertung_ISS/data/007_2018-07-04_16-44-22/raw_I005_X1_C3.fits.SIM.fits", path "E:/Auswertung_ISS/data/007_2018-07-04_16-44-22/raw_I006_X1_C0.fits.SIM.fits", path "E:/Auswertung_ISS/data/007_2018-07-04_16-44-22/raw_I006_X1_C3.fits.SIM.fits", path "E:/Auswertung_ISS/data/007_2018-07-04_16-44-22/raw_I007_X1_C0.fits.SIM.fits", path "E:/Auswertung_ISS/data/007_2018-07-04_16-44-22/raw_I007_X1_C3.fits.SIM.fits", path "E:/Auswertung_ISS/data/007_2018-07-04_16-44-22/raw_I008_X1_C0.fits.SIM.fits", path "E:/Auswertung_ISS/data/007_2018-07-04_16-44-22/raw_I008_X1_C3.fits.SIM.fits", path "E:/Auswertung_ISS/data/007_2018-07-04_16-44-22/raw_I008_X1_C3.fits.simpleSIM.fits", path "E:/Auswertung_ISS/data/007_2018-07-04_16-44-22/raw_I009_X1_C0.fits.SIM.fits", path "E:/Auswertung_ISS/data/007_2018-07-04_16-44-22/raw_I009_X1_C3.fits.SIM.fits", path "E:/Auswertung_ISS/data/007_2018-07-04_16-44-22/raw_I010_X1_C0.fits.SIM.fits", path "E:/Auswertung_ISS/data/007_2018-07-04_16-44-22/raw_I010_X1_C3.fits.SIM.fits", path "E:/Auswertung_ISS/data/007_2018-07-04_16-44-22/raw_I011_X1_C0.fits.SIM.fits", path "E:/Auswertung_ISS/data/007_2018-07-04_16-44-22/raw_I011_X1_C3.fits.SIM.fits", path "E:/Auswertung_ISS/data/007_2018-07-04_16-44-22/raw_I012_X1_C0.fits.SIM.fits", path "E:/Auswertung_ISS/data/007_2018-07-04_16-44-22/raw_I012_X1_C3.fits.SIM.fits", path "E:/Auswertung_ISS/data/007_2018-07-04_16-44-22/raw_I013_X1_C0.fits.SIM.fits", path "E:/Auswertung_ISS/data/007_2018-07-04_16-44-22/raw_I013_X1_C3.fits.SIM.fits", path "E:/Auswertung_ISS/data/007_2018-07-04_16-44-22/raw_I014_X1_C0.fits.SIM.fits", path "E:/Auswertung_ISS/data/007_2018-07-04_16-44-22/raw_I014_X1_C3.fits.SIM.fits", path "E:/Auswertung_ISS/data/007_2018-07-04_16-44-22/raw_I015_X1_C0.fits.SIM.fits", path "E:/Auswertung_ISS/data/007_2018-07-04_16-44-22/raw_I015_X1_C3.fits.SIM.fits", path "E:/Auswertung_ISS/data/007_2018-07-04_16-44-22/raw_I016_X1_C0.fits.SIM.fits", path "E:/Auswertung_ISS/data/007_2018-07-04_16-44-22/raw_I016_X1_C3.fits.SIM.fits", path "E:/Auswertung_ISS/data/007_2018-07-04_16-44-22/raw_I017_X1_C0.fits.SIM.fits", path "E:/Auswertung_ISS/data/007_2018-07-04_16-44-22/raw_I017_X1_C3.fits.SIM.fits", path "E:/Auswertung_ISS/data/008_2018-07-05_08-02-52/raw_I000_X0_C0.fits.SIM.fits", path "E:/Auswertung_ISS/data/008_2018-07-05_08-02-52/raw_I000_X0_C1.fits.SIM.fits", path "E:/Auswertung_ISS/data/008_2018-07-05_08-02-52/raw_I000_X0_C3.fits.SIM.fits", path "E:/Auswertung_ISS/data/008_2018-07-05_08-02-52/raw_I000_X1_C0.fits.SIM.fits", path "E:/Auswertung_ISS/data/008_2018-07-05_08-02-52/raw_I000_X1_C3.fits.SIM.fits", path "E:/Auswertung_ISS/data/008_2018-07-05_08-02-52/raw_I001_X1_C0.fits.SIM.fits", path "E:/Auswertung_ISS/data/008_2018-07-05_08-02-52/raw_I001_X1_C3.fits.SIM.fits", path "E:/Auswertung_ISS/data/008_2018-07-05_08-02-52/raw_I002_X1_C0.fits.SIM.fits", path "E:/Auswertung_ISS/data/008_2018-07-05_08-02-52/raw_I002_X1_C3.fits.SIM.fits", path "E:/Auswertung_ISS/data/008_2018-07-05_08-02-52/raw_I003_X1_C0.fits.SIM.fits", path "E:/Auswertung_ISS/data/008_2018-07-05_08-02-52/raw_I003_X1_C3.fits.SIM.fits", path "E:/Auswertung_ISS/data/008_2018-07-05_08-02-52/raw_I004_X1_C0.fits.SIM.fits", path "E:/Auswertung_ISS/data/008_2018-07-05_08-02-52/raw_I004_X1_C3.fits.SIM.fits", path "E:/Auswertung_ISS/data/008_2018-07-05_08-02-52/raw_I005_X1_C0.fits.SIM.fits", path "E:/Auswertung_ISS/data/008_2018-07-05_08-02-52/raw_I005_X1_C3.fits.SIM.fits", path "E:/Auswertung_ISS/data/008_2018-07-05_08-02-52/raw_I006_X1_C0.fits.SIM.fits", path "E:/Auswertung_ISS/data/008_2018-07-05_08-02-52/raw_I006_X1_C3.fits.SIM.fits", path "E:/Auswertung_ISS/data/008_2018-07-05_08-02-52/raw_I007_X1_C0.fits.SIM.fits", path "E:/Auswertung_ISS/data/008_2018-07-05_08-02-52/raw_I007_X1_C3.fits.SIM.fits", path "E:/Auswertung_ISS/data/008_2018-07-05_08-02-52/raw_I008_X1_C0.fits.SIM.fits", path "E:/Auswertung_ISS/data/008_2018-07-05_08-02-52/raw_I008_X1_C3.fits.SIM.fits", path "E:/Auswertung_ISS/data/008_2018-07-05_08-02-52/raw_I009_X1_C0.fits.SIM.fits", path "E:/Auswertung_ISS/data/008_2018-07-05_08-02-52/raw_I009_X1_C3.fits.SIM.fits", path "E:/Auswertung_ISS/data/008_2018-07-05_08-02-52/raw_I010_X1_C0.fits.SIM.fits", path "E:/Auswertung_ISS/data/008_2018-07-05_08-02-52/raw_I010_X1_C3.fits.SIM.fits", path "E:/Auswertung_ISS/data/008_2018-07-05_08-02-52/raw_I011_X1_C0.fits.SIM.fits", path "E:/Auswertung_ISS/data/008_2018-07-05_08-02-52/raw_I011_X1_C3.fits.SIM.fits", path "E:/Auswertung_ISS/data/008_2018-07-05_08-02-52/raw_I012_X1_C0.fits.SIM.fits", path "E:/Auswertung_ISS/data/008_2018-07-05_08-02-52/raw_I012_X1_C3.fits.SIM.fits", path "E:/Auswertung_ISS/data/008_2018-07-05_08-02-52/raw_I013_X1_C0.fits.SIM.fits", path "E:/Auswertung_ISS/data/008_2018-07-05_08-02-52/raw_I013_X1_C3.fits.SIM.fits", path "E:/Auswertung_ISS/data/008_2018-07-05_08-02-52/raw_I014_X1_C0.fits.SIM.fits", path "E:/Auswertung_ISS/data/008_2018-07-05_08-02-52/raw_I014_X1_C3.fits.SIM.fits", path "E:/Auswertung_ISS/data/008_2018-07-05_08-02-52/raw_I015_X1_C0.fits.SIM.fits", path "E:/Auswertung_ISS/data/008_2018-07-05_08-02-52/raw_I015_X1_C3.fits.SIM.fits", path "E:/Auswertung_ISS/data/008_2018-07-05_08-02-52/raw_I016_X1_C0.fits.SIM.fits", path "E:/Auswertung_ISS/data/008_2018-07-05_08-02-52/raw_I016_X1_C3.fits.SIM.fits", path "E:/Auswertung_ISS/data/008_2018-07-05_08-02-52/raw_I017_X1_C0.fits.SIM.fits", path "E:/Auswertung_ISS/data/008_2018-07-05_08-02-52/raw_I017_X1_C3.fits.SIM.fits", path "E:/Auswertung_ISS/data/009_2018-07-05_20-57-36/raw_I000_X0_C0.fits.SIM.fits", path "E:/Auswertung_ISS/data/009_2018-07-05_20-57-36/raw_I000_X0_C1.fits.SIM.fits", path "E:/Auswertung_ISS/data/009_2018-07-05_20-57-36/raw_I000_X0_C3.fits.SIM.fits", path "E:/Auswertung_ISS/data/009_2018-07-05_20-57-36/raw_I000_X1_C3.fits.SIM.fits", path "E:/Auswertung_ISS/data/009_2018-07-05_20-57-36/raw_I001_X1_C3.fits.SIM.fits", path "E:/Auswertung_ISS/data/009_2018-07-05_20-57-36/raw_I002_X1_C3.fits.SIM.fits", path "E:/Auswertung_ISS/data/009_2018-07-05_20-57-36/raw_I003_X1_C3.fits.SIM.fits", path "E:/Auswertung_ISS/data/009_2018-07-05_20-57-36/raw_I004_X1_C3.fits.SIM.fits", path "E:/Auswertung_ISS/data/009_2018-07-05_20-57-36/raw_I005_X1_C3.fits.SIM.fits", path "E:/Auswertung_ISS/data/009_2018-07-05_20-57-36/raw_I006_X1_C3.fits.SIM.fits", path "E:/Auswertung_ISS/data/009_2018-07-05_20-57-36/raw_I007_X1_C3.fits.SIM.fits", path "E:/Auswertung_ISS/data/009_2018-07-05_20-57-36/raw_I008_X1_C3.fits.SIM.fits", path "E:/Auswertung_ISS/data/009_2018-07-05_20-57-36/raw_I009_X1_C3.fits.SIM.fits", path "E:/Auswertung_ISS/data/009_2018-07-05_20-57-36/raw_I010_X1_C3.fits.SIM.fits", path "E:/Auswertung_ISS/data/009_2018-07-05_20-57-36/raw_I011_X1_C3.fits.SIM.fits", path "E:/Auswertung_ISS/data/010_2018-07-06_17-20-26/raw_I000_X0_C0.fits.SIM.fits", path "E:/Auswertung_ISS/data/010_2018-07-06_17-20-26/raw_I000_X0_C1.fits.SIM.fits", path "E:/Auswertung_ISS/data/010_2018-07-06_17-20-26/raw_I000_X0_C3.fits.SIM.fits", path "E:/Auswertung_ISS/data/010_2018-07-06_17-20-26/raw_I000_X1_C3.fits.SIM.fits", path "E:/Auswertung_ISS/data/010_2018-07-06_17-20-26/raw_I001_X0_C0.fits.SIM.fits", path "E:/Auswertung_ISS/data/010_2018-07-06_17-20-26/raw_I001_X0_C1.fits.SIM.fits", path "E:/Auswertung_ISS/data/010_2018-07-06_17-20-26/raw_I001_X0_C3.fits.SIM.fits", path "E:/Auswertung_ISS/data/011_2018-07-06_17-40-54/raw_I000_X0_C0.fits.SIM.fits", path "E:/Auswertung_ISS/data/011_2018-07-06_17-40-54/raw_I000_X0_C1.fits.SIM.fits", path "E:/Auswertung_ISS/data/011_2018-07-06_17-40-54/raw_I000_X0_C3.fits.SIM.fits", path "E:/Auswertung_ISS/data/011_2018-07-06_17-40-54/raw_I000_X1_C3.fits.SIM.fits", path "E:/Auswertung_ISS/data/011_2018-07-06_17-40-54/raw_I001_X1_C3.fits.SIM.fits", path "E:/Auswertung_ISS/data/011_2018-07-06_17-40-54/raw_I002_X1_C3.fits.SIM.fits", path "E:/Auswertung_ISS/data/011_2018-07-06_17-40-54/raw_I003_X1_C3.fits.SIM.fits", path "E:/Auswertung_ISS/data/011_2018-07-06_17-40-54/raw_I004_X1_C3.fits.SIM.fits", path "E:/Auswertung_ISS/data/011_2018-07-06_17-40-54/raw_I005_X1_C3.fits.SIM.fits", path "E:/Auswertung_ISS/data/011_2018-07-06_17-40-54/raw_I006_X1_C3.fits.SIM.fits", path "E:/Auswertung_ISS/data/011_2018-07-06_17-40-54/raw_I007_X1_C3.fits.SIM.fits", path "E:/Auswertung_ISS/data/011_2018-07-06_17-40-54/raw_I008_X1_C3.fits.SIM.fits", path "E:/Auswertung_ISS/data/012_2018-07-07_01-02-54/raw_I000_X0_C0.fits.SIM.fits", path "E:/Auswertung_ISS/data/012_2018-07-07_01-02-54/raw_I000_X0_C1.fits.SIM.fits", path "E:/Auswertung_ISS/data/012_2018-07-07_01-02-54/raw_I000_X0_C3.fits.SIM.fits", path "E:/Auswertung_ISS/data/012_2018-07-07_01-02-54/raw_I000_X1_C3.fits.SIM.fits", path "E:/Auswertung_ISS/data/012_2018-07-07_01-02-54/raw_I001_X1_C3.fits.SIM.fits", path "E:/Auswertung_ISS/data/012_2018-07-07_01-02-54/raw_I002_X1_C3.fits.SIM.fits", path "E:/Auswertung_ISS/data/012_2018-07-07_01-02-54/raw_I003_X1_C3.fits.SIM.fits", path "E:/Auswertung_ISS/data/012_2018-07-07_01-02-54/raw_I004_X1_C3.fits.SIM.fits", path "E:/Auswertung_ISS/data/012_2018-07-07_01-02-54/raw_I005_X1_C3.fits.SIM.fits", path "E:/Auswertung_ISS/data/012_2018-07-07_01-02-54/raw_I006_X1_C3.fits.SIM.fits", path "E:/Auswertung_ISS/data/013_2018-07-07_08-02-53/raw_I000_X0_C0.fits.SIM.fits", path "E:/Auswertung_ISS/data/013_2018-07-07_08-02-53/raw_I000_X0_C1.fits.SIM.fits", path "E:/Auswertung_ISS/data/013_2018-07-07_08-02-53/raw_I000_X0_C3.fits.SIM.fits", path "E:/Auswertung_ISS/data/013_2018-07-07_08-02-53/raw_I000_X1_C0.fits.SIM.fits", path "E:/Auswertung_ISS/data/013_2018-07-07_08-02-53/raw_I000_X1_C3.fits.SIM.fits", path "E:/Auswertung_ISS/data/013_2018-07-07_08-02-53/raw_I001_X1_C0.fits.SIM.fits", path "E:/Auswertung_ISS/data/013_2018-07-07_08-02-53/raw_I001_X1_C3.fits.SIM.fits", path "E:/Auswertung_ISS/data/013_2018-07-07_08-02-53/raw_I002_X1_C0.fits.SIM.fits", path "E:/Auswertung_ISS/data/013_2018-07-07_08-02-53/raw_I002_X1_C3.fits.SIM.fits", path "E:/Auswertung_ISS/data/013_2018-07-07_08-02-53/raw_I003_X1_C0.fits.SIM.fits", path "E:/Auswertung_ISS/data/013_2018-07-07_08-02-53/raw_I003_X1_C3.fits.SIM.fits", path "E:/Auswertung_ISS/data/013_2018-07-07_08-02-53/raw_I004_X1_C0.fits.SIM.fits", path "E:/Auswertung_ISS/data/013_2018-07-07_08-02-53/raw_I004_X1_C3.fits.SIM.fits", path "E:/Auswertung_ISS/data/013_2018-07-07_08-02-53/raw_I005_X1_C0.fits.SIM.fits", path "E:/Auswertung_ISS/data/013_2018-07-07_08-02-53/raw_I005_X1_C3.fits.SIM.fits", path "E:/Auswertung_ISS/data/013_2018-07-07_08-02-53/raw_I006_X1_C0.fits.SIM.fits", path "E:/Auswertung_ISS/data/013_2018-07-07_08-02-53/raw_I006_X1_C3.fits.SIM.fits", path "E:/Auswertung_ISS/data/013_2018-07-07_08-02-53/raw_I007_X1_C0.fits.SIM.fits", path "E:/Auswertung_ISS/data/013_2018-07-07_08-02-53/raw_I007_X1_C3.fits.SIM.fits", path "E:/Auswertung_ISS/data/013_2018-07-07_08-02-53/raw_I008_X1_C0.fits.SIM.fits", path "E:/Auswertung_ISS/data/013_2018-07-07_08-02-53/raw_I008_X1_C3.fits.SIM.fits", path "E:/Auswertung_ISS/data/013_2018-07-07_08-02-53/raw_I009_X1_C0.fits.SIM.fits", path "E:/Auswertung_ISS/data/013_2018-07-07_08-02-53/raw_I009_X1_C3.fits.SIM.fits", path "E:/Auswertung_ISS/data/013_2018-07-07_08-02-53/raw_I010_X1_C0.fits.SIM.fits", path "E:/Auswertung_ISS/data/013_2018-07-07_08-02-53/raw_I010_X1_C3.fits.SIM.fits", path "E:/Auswertung_ISS/data/013_2018-07-07_08-02-53/raw_I011_X1_C0.fits.SIM.fits", path "E:/Auswertung_ISS/data/013_2018-07-07_08-02-53/raw_I011_X1_C3.fits.SIM.fits", path "E:/Auswertung_ISS/data/013_2018-07-07_08-02-53/raw_I012_X1_C0.fits.SIM.fits", path "E:/Auswertung_ISS/data/013_2018-07-07_08-02-53/raw_I012_X1_C3.fits.SIM.fits", path "E:/Auswertung_ISS/data/013_2018-07-07_08-02-53/raw_I013_X1_C0.fits.SIM.fits", path "E:/Auswertung_ISS/data/013_2018-07-07_08-02-53/raw_I013_X1_C3.fits.SIM.fits", path "E:/Auswertung_ISS/data/013_2018-07-07_08-02-53/raw_I014_X1_C0.fits.SIM.fits", path "E:/Auswertung_ISS/data/013_2018-07-07_08-02-53/raw_I014_X1_C3.fits.SIM.fits", path "E:/Auswertung_ISS/data/013_2018-07-07_08-02-53/raw_I015_X1_C0.fits.SIM.fits", path "E:/Auswertung_ISS/data/013_2018-07-07_08-02-53/raw_I015_X1_C3.fits.SIM.fits", path "E:/Auswertung_ISS/data/013_2018-07-07_08-02-53/raw_I016_X1_C0.fits.SIM.fits", path "E:/Auswertung_ISS/data/013_2018-07-07_08-02-53/raw_I016_X1_C3.fits.SIM.fits", path "E:/Auswertung_ISS/data/013_2018-07-07_08-02-53/raw_I017_X1_C0.fits.SIM.fits", path "E:/Auswertung_ISS/data/013_2018-07-07_08-02-53/raw_I017_X1_C3.fits.SIM.fits", path "E:/Auswertung_ISS/data/013_2018-07-07_08-02-53/raw_I018_X1_C0.fits.SIM.fits", path "E:/Auswertung_ISS/data/013_2018-07-07_08-02-53/raw_I018_X1_C3.fits.SIM.fits", path "E:/Auswertung_ISS/data/013_2018-07-07_08-02-53/raw_I019_X1_C0.fits.SIM.fits", path "E:/Auswertung_ISS/data/013_2018-07-07_08-02-53/raw_I019_X1_C3.fits.SIM.fits", path "E:/Auswertung_ISS/data/013_2018-07-07_08-02-53/raw_I020_X1_C0.fits.SIM.fits", path "E:/Auswertung_ISS/data/013_2018-07-07_08-02-53/raw_I020_X1_C3.fits.SIM.fits", path "E:/Auswertung_ISS/data/013_2018-07-07_08-02-53/raw_I021_X1_C0.fits.SIM.fits", path "E:/Auswertung_ISS/data/013_2018-07-07_08-02-53/raw_I021_X1_C3.fits.SIM.fits", path "E:/Auswertung_ISS/data/013_2018-07-07_08-02-53/raw_I022_X1_C0.fits.SIM.fits", path "E:/Auswertung_ISS/data/013_2018-07-07_08-02-53/raw_I022_X1_C3.fits.SIM.fits", path "E:/Auswertung_ISS/data/013_2018-07-07_08-02-53/raw_I023_X1_C0.fits.SIM.fits", path "E:/Auswertung_ISS/data/013_2018-07-07_08-02-53/raw_I023_X1_C3.fits.SIM.fits", path "E:/Auswertung_ISS/data/013_2018-07-07_08-02-53/raw_I024_X1_C0.fits.SIM.fits", path "E:/Auswertung_ISS/data/013_2018-07-07_08-02-53/raw_I024_X1_C3.fits.SIM.fits", path "E:/Auswertung_ISS/data/013_2018-07-07_08-02-53/raw_I025_X1_C0.fits.SIM.fits", path "E:/Auswertung_ISS/data/013_2018-07-07_08-02-53/raw_I025_X1_C3.fits.SIM.fits", path "E:/Auswertung_ISS/data/013_2018-07-07_08-02-53/raw_I026_X1_C0.fits.SIM.fits", path "E:/Auswertung_ISS/data/013_2018-07-07_08-02-53/raw_I026_X1_C3.fits.SIM.fits", path "E:/Auswertung_ISS/data/013_2018-07-07_08-02-53/raw_I027_X1_C0.fits.SIM.fits", path "E:/Auswertung_ISS/data/013_2018-07-07_08-02-53/raw_I027_X1_C3.fits.SIM.fits", path "E:/Auswertung_ISS/data/013_2018-07-07_08-02-53/raw_I028_X1_C0.fits.SIM.fits", path "E:/Auswertung_ISS/data/013_2018-07-07_08-02-53/raw_I028_X1_C3.fits.SIM.fits", path "E:/Auswertung_ISS/data/013_2018-07-07_08-02-53/raw_I029_X1_C0.fits.SIM.fits", path "E:/Auswertung_ISS/data/013_2018-07-07_08-02-53/raw_I029_X1_C3.fits.SIM.fits", path "E:/Auswertung_ISS/data/014_2018-07-16_17-53-52/raw_I000_X0_C0.fits.SIM.fits", path "E:/Auswertung_ISS/data/014_2018-07-16_17-53-52/raw_I000_X0_C1.fits.SIM.fits", path "E:/Auswertung_ISS/data/014_2018-07-16_17-53-52/raw_I000_X0_C3.fits.SIM.fits", path "E:/Auswertung_ISS/data/014_2018-07-16_17-53-52/raw_I000_X1_C0.fits.SIM.fits", path "E:/Auswertung_ISS/data/014_2018-07-16_17-53-52/raw_I000_X1_C3.fits.SIM.fits", path "E:/Auswertung_ISS/data/014_2018-07-16_17-53-52/raw_I001_X1_C0.fits.SIM.fits", path "E:/Auswertung_ISS/data/014_2018-07-16_17-53-52/raw_I001_X1_C3.fits.SIM.fits", path "E:/Auswertung_ISS/data/014_2018-07-16_17-53-52/raw_I002_X1_C0.fits.SIM.fits", path "E:/Auswertung_ISS/data/014_2018-07-16_17-53-52/raw_I002_X1_C3.fits.SIM.fits", path "E:/Auswertung_ISS/data/014_2018-07-16_17-53-52/raw_I003_X1_C0.fits.SIM.fits", path "E:/Auswertung_ISS/data/014_2018-07-16_17-53-52/raw_I003_X1_C3.fits.SIM.fits", path "E:/Auswertung_ISS/data/014_2018-07-16_17-53-52/raw_I004_X1_C0.fits.SIM.fits", path "E:/Auswertung_ISS/data/014_2018-07-16_17-53-52/raw_I004_X1_C3.fits.SIM.fits", path "E:/Auswertung_ISS/data/014_2018-07-16_17-53-52/raw_I005_X1_C0.fits.SIM.fits", path "E:/Auswertung_ISS/data/014_2018-07-16_17-53-52/raw_I005_X1_C3.fits.SIM.fits", path "E:/Auswertung_ISS/data/014_2018-07-16_17-53-52/raw_I006_X1_C0.fits.SIM.fits", path "E:/Auswertung_ISS/data/014_2018-07-16_17-53-52/raw_I006_X1_C3.fits.SIM.fits", path "E:/Auswertung_ISS/data/014_2018-07-16_17-53-52/raw_I007_X1_C0.fits.SIM.fits", path "E:/Auswertung_ISS/data/014_2018-07-16_17-53-52/raw_I007_X1_C3.fits.SIM.fits", path "E:/Auswertung_ISS/data/014_2018-07-16_17-53-52/raw_I008_X1_C0.fits.SIM.fits", path "E:/Auswertung_ISS/data/014_2018-07-16_17-53-52/raw_I008_X1_C3.fits.SIM.fits", path "E:/Auswertung_ISS/data/014_2018-07-16_17-53-52/raw_I009_X1_C0.fits.SIM.fits", path "E:/Auswertung_ISS/data/014_2018-07-16_17-53-52/raw_I009_X1_C3.fits.SIM.fits", path "E:/Auswertung_ISS/data/014_2018-07-16_17-53-52/raw_I010_X1_C0.fits.SIM.fits", path "E:/Auswertung_ISS/data/014_2018-07-16_17-53-52/raw_I010_X1_C3.fits.SIM.fits", path "E:/Auswertung_ISS/data/014_2018-07-16_17-53-52/raw_I011_X1_C0.fits.SIM.fits", path "E:/Auswertung_ISS/data/014_2018-07-16_17-53-52/raw_I011_X1_C3.fits.SIM.fits", path "E:/Auswertung_ISS/data/014_2018-07-16_17-53-52/raw_I012_X1_C0.fits.SIM.fits", path "E:/Auswertung_ISS/data/014_2018-07-16_17-53-52/raw_I012_X1_C3.fits.SIM.fits", path "E:/Auswertung_ISS/data/014_2018-07-16_17-53-52/raw_I013_X1_C0.fits.SIM.fits", path "E:/Auswertung_ISS/data/014_2018-07-16_17-53-52/raw_I013_X1_C3.fits.SIM.fits", path "E:/Auswertung_ISS/data/014_2018-07-16_17-53-52/raw_I014_X1_C0.fits.SIM.fits", path "E:/Auswertung_ISS/data/014_2018-07-16_17-53-52/raw_I014_X1_C3.fits.SIM.fits", path "E:/Auswertung_ISS/data/014_2018-07-16_17-53-52/raw_I015_X1_C0.fits.SIM.fits", path "E:/Auswertung_ISS/data/014_2018-07-16_17-53-52/raw_I015_X1_C3.fits.SIM.fits", path "E:/Auswertung_ISS/data/014_2018-07-16_17-53-52/raw_I016_X1_C0.fits.SIM.fits", path "E:/Auswertung_ISS/data/014_2018-07-16_17-53-52/raw_I016_X1_C3.fits.SIM.fits", path "E:/Auswertung_ISS/data/014_2018-07-16_17-53-52/raw_I017_X1_C0.fits.SIM.fits", path "E:/Auswertung_ISS/data/014_2018-07-16_17-53-52/raw_I017_X1_C3.fits.SIM.fits", path "E:/Auswertung_ISS/data/014_2018-07-16_17-53-52/raw_I018_X1_C0.fits.SIM.fits", path "E:/Auswertung_ISS/data/014_2018-07-16_17-53-52/raw_I018_X1_C3.fits.SIM.fits", path "E:/Auswertung_ISS/data/014_2018-07-16_17-53-52/raw_I019_X1_C0.fits.SIM.fits", path "E:/Auswertung_ISS/data/014_2018-07-16_17-53-52/raw_I019_X1_C3.fits.SIM.fits", path "E:/Auswertung_ISS/data/014_2018-07-16_17-53-52/raw_I020_X1_C0.fits.SIM.fits", path "E:/Auswertung_ISS/data/014_2018-07-16_17-53-52/raw_I020_X1_C3.fits.SIM.fits", path "E:/Auswertung_ISS/data/014_2018-07-16_17-53-52/raw_I021_X1_C0.fits.SIM.fits", path "E:/Auswertung_ISS/data/014_2018-07-16_17-53-52/raw_I021_X1_C3.fits.SIM.fits", path "E:/Auswertung_ISS/data/014_2018-07-16_17-53-52/raw_I022_X1_C0.fits.SIM.fits", path "E:/Auswertung_ISS/data/014_2018-07-16_17-53-52/raw_I022_X1_C3.fits.SIM.fits", path "E:/Auswertung_ISS/data/014_2018-07-16_17-53-52/raw_I023_X1_C0.fits.SIM.fits", path "E:/Auswertung_ISS/data/014_2018-07-16_17-53-52/raw_I023_X1_C3.fits.SIM.fits", path "E:/Auswertung_ISS/data/014_2018-07-16_17-53-52/raw_I024_X1_C0.fits.SIM.fits", path "E:/Auswertung_ISS/data/014_2018-07-16_17-53-52/raw_I024_X1_C3.fits.SIM.fits", path "E:/Auswertung_ISS/data/014_2018-07-16_17-53-52/raw_I025_X1_C0.fits.SIM.fits", path "E:/Auswertung_ISS/data/014_2018-07-16_17-53-52/raw_I025_X1_C3.fits.SIM.fits", path "E:/Auswertung_ISS/data/014_2018-07-16_17-53-52/raw_I026_X1_C0.fits.SIM.fits", path "E:/Auswertung_ISS/data/014_2018-07-16_17-53-52/raw_I026_X1_C3.fits.SIM.fits", path "E:/Auswertung_ISS/data/014_2018-07-16_17-53-52/raw_I027_X1_C0.fits.SIM.fits", path "E:/Auswertung_ISS/data/014_2018-07-16_17-53-52/raw_I027_X1_C3.fits.SIM.fits", path "E:/Auswertung_ISS/data/014_2018-07-16_17-53-52/raw_I028_X1_C0.fits.SIM.fits", path "E:/Auswertung_ISS/data/014_2018-07-16_17-53-52/raw_I028_X1_C3.fits.SIM.fits", path "E:/Auswertung_ISS/data/014_2018-07-16_17-53-52/raw_I029_X1_C0.fits.SIM.fits", path "E:/Auswertung_ISS/data/014_2018-07-16_17-53-52/raw_I029_X1_C3.fits.SIM.fits"]
  # "use Recusrive File List"
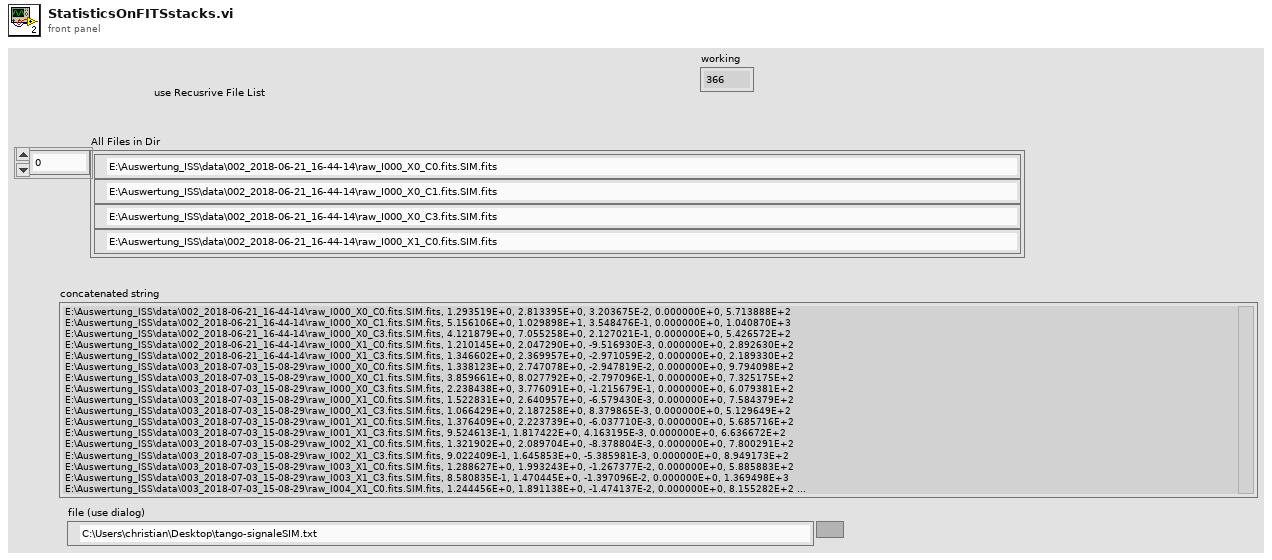
[diagram p1: front panel]
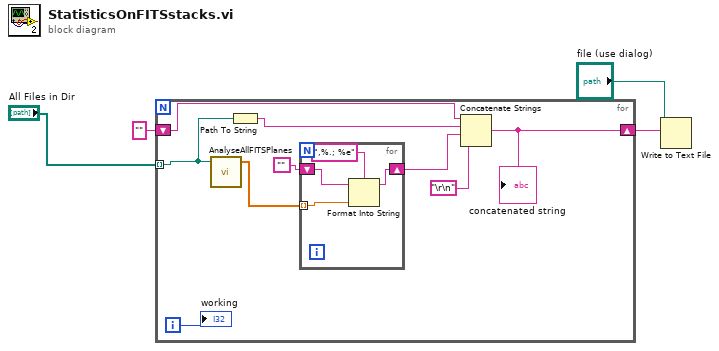
[diagram p0: block diagram]
diagram:
  n1 = for {
    tunnel: "All Files in Dir" -> [w12] mode=indexing
    shift-right: [w7] -> w2
    shift-left: "" -> [w5]
    i -> [w13]
    n2 = call "AnalyseAllFITSPlanes.vi"("file path"=w12) -> ("Mean,std,slope,min,max"=w11:dbl[])  [unwired: 3 in, 1 out]
    n3 = Path To String(path=w12) -> (string=w9:string)
    n4 = for {
      tunnel: w11 -> [w17] mode=indexing
      shift-right: [w16] -> w8
      shift-left: "" -> [w14]
      n5 = Format Into String(format string=",%.; %e", initial string=w14, w17) -> (resulting string=w16:string)  [unwired: 1 in, 1 out]
    }
    n6 = Concatenate Strings(w5, w9, w8, "\r\n") -> (w7:string)
    "concatenated string" <- w7
    "working" <- w13
  }
  n7 = Write to Text File(file (use dialog)="file (use dialog)", text=w2) -> ()  [unwired: 2 in, 3 out]
